vi "GESTIONE FRENO.vi"(10 "Sub Panel freno":refnum<vi>) -> ()   [LabVIEW 2019]
uses:
  TypeDef/InverterFreno.ctl
  TypeDef/Stato_inverter.ctl
  TypeDef/Comandi freno.ctl
  TypeDef/Stato inverter selezionato.ctl
  cDAQ_PLC Folder/cDAQ/SET SINGLE DO.ctl
  cDAQ_PLC Folder/cDAQ/DO List.ctl
  cDAQ_PLC Folder/cDAQ/SET SINGLE AO.ctl
  cDAQ_PLC Folder/cDAQ/AO List.ctl
  BenchSelector.vi
  Global_All_Data.vi
  Stato alimentatore 1.vi
  Global control type freno.vi
  Stato comandi freno.vi
  Global CAMBIO CTRL FRENO.vi
  Global FINE AVVIO.vi
  Fine rampa sinus penta.vi
  Global Trampa 0.vi
  Global CTRL VELOCITA.vi
  cDAQ_PLC Folder/cDAQ/SET ARRAY DO.ctl
  Global senso rotazione.vi
  <vilib>/Utility/file.llb/Read Delimited Spreadsheet (string).vi
panel:
  out "A max":dbl
  out "Freno selezionato":i32
  out "Rpm max":dbl
  out "Cmax":dbl
  out "KW max Banco 1":dbl
  out "KW max Banco 2":dbl
  out "RPM max Banco 1":dbl
  out "RPM max Banco 2":dbl
  out "A max Banco 2":dbl
  out "A max Banco 1":dbl
  out "Nm max Banco 2":dbl
  out "Nm max Banco 1":dbl
  out "all rows":string[][](array[string])
  out "Comandi freno":T1[](array[typedef]) {"Rif AO coppia freno[Nm]" format="%#_13g"}
  out "Array stato inverter freno":T1[](array[typedef]) {"Rif AO coppia freno[Nm]" format="%#_13g"}
  in  "rif vel":bool
  in  "Rif % AO RPM":dbl
  out "# elements in queue":i32
  out "DO senso rotaz freno":bool=TRUE
  out "Rpm stabile":bool
  out "Ctrl coppia":bool
  out "Ctrl velocità":bool
  in  "simula?":bool
  out "KW max banco":dbl
  out "Kw Max prova":dbl
  out "INVERTI SENSO ROT":bool
  out "DI senso rotaz freno":bool
  out "Message":string
  out "Abilita":bool=TRUE
  out "fine rampa C":bool
  out "fine rampa rpm":bool
  out "P Stabile?":bool
  out "start":bool=TRUE
  out "Controllo desiderato":T2(ring)
  out "Controllo effettivo":T2(ring)
  out "C Stabile?":bool
  out "Rif AO coppia freno [Nm]":dbl format="%#_13g"
  out "Rif AO vel [RPM]":dbl
  in  "Precisione pid Nm":dbl caption="Nm"
  in  "Precisione pid W":dbl caption="W"
  out "Boolean 2":bool
  in  "Compensazione velocità":bool=TRUE
  out "Comp.":bool
  in  "Gestione freno":T3 {"Status ref"."Speed" max=2000.0; "Status ref"."Torque" max=2000.0; "Control"."Set" min=0.0 max=0.0 format="%#.2f"}
  out "C->rpm":string
  out "rpm->C":string
  out "Boolean":bool
  in  "OK Button":bool
  out "Stato comandi":T3
  in  "Salva config freni":bool
  in  "rpm":dbl
  in  "x":dbl
  in  "stop":bool
  in  "ARRAY IMPOSTAZIONI INV.FRENI":T4[](array[typedef])=[{"Nome"="", "Cmax"=100.0, "Rpm max"=3000.0, "A max"=0.0, "Controllo RPM"={"PID gains Rpm"={"proportional gain (Kc)"=0.0, "integral time (Ti, min)"=0.0, "derivative time (Td, min)"=0.0}, "Abilita pid"=FALSE, "Precisione pid Rpm"=0.015, "Medie pid"=10, "Trampa[s]"=10, "Tstab ramp[s]"=10, "Max%pid"=10}, "Controllo coppia"={"PID gains Coppia"={"proportional gain (Kc)"=10.0, "integral time (Ti, min)"=0.015, "derivative time (Td, min)"=0.0}, "Abilita pid"=FALSE, "Precisione pid Nm"=0.0, "Medie pid"=0, "Trampa[s]"=0, "Tstab ramp[s]"=10, "Max%pid"=10}, "Controllo potenza"={"PID gains potenza"={"proportional gain (Kc)"=0.4, "integral time (Ti, min)"=0.025, "derivative time (Td, min)"=0.0}, "Abilita pid"=FALSE, "Precisione pid W"=0.015, "Medie pid"=10, "Trampa[s]"=10, "Tstab ramp[s]"=10, "Max%pid"=10}, "Compensa coppia residua"={"Abilita compensazione"=FALSE, "C residua [Nm]"=0.0, "C isteresi [Nm]"=0.0, "PID gains C-RPM"={"proportional gain (Kc)"=1.0, "integral time (Ti, min)"=0.01, "derivative time (Td, min)"=0.0}, "C precision [Nm]"=0.0, "Max%pid"=0, "Medie pid"=0}}, {"Nome"="", "Cmax"=200.0, "Rpm max"=4500.0, "A max"=0.0, "Controllo RPM"={"PID gains Rpm"={"proportional gain (Kc)"=0.0, "integral time (Ti, min)"=0.0, "derivative time (Td, min)"=0.0}, "Abilita pid"=FALSE, "Precisione pid Rpm"=0.015, "Medie pid"=10, "Trampa[s]"=10, "Tstab ramp[s]"=10, "Max%pid"=10}, "Controllo coppia"={"PID gains Coppia"={"proportional gain (Kc)"=10.0, "integral time (Ti, min)"=0.015, "derivative time (Td, min)"=0.0}, "Abilita pid"=FALSE, "Precisione pid Nm"=0.0, "Medie pid"=0, "Trampa[s]"=0, "Tstab ramp[s]"=10, "Max%pid"=10}, "Controllo potenza"={"PID gains potenza"={"proportional gain (Kc)"=0.4, "integral time (Ti, min)"=0.025, "derivative time (Td, min)"=0.0}, "Abilita pid"=FALSE, "Precisione pid W"=0.015, "Medie pid"=10, "Trampa[s]"=10, "Tstab ramp[s]"=10, "Max%pid"=10}, "Compensa coppia residua"={"Abilita compensazione"=FALSE, "C residua [Nm]"=0.0, "C isteresi [Nm]"=0.0, "PID gains C-RPM"={"proportional gain (Kc)"=1.0, "integral time (Ti, min)"=0.01, "derivative time (Td, min)"=0.0}, "C precision [Nm]"=0.0, "Max%pid"=0, "Medie pid"=0}}] {"Controllo RPM"."Precisione pid Rpm" format="%#_13g"; "Controllo RPM"."PID gains Rpm"."derivative time (Td, min)" format="%.3f"; "Controllo RPM"."PID gains Rpm"."integral time (Ti, min)" format="%.3f"; "Controllo RPM"."PID gains Rpm"."proportional gain (Kc)" format="%.3f"; "Controllo potenza"."Precisione pid W" format="%#_13g"; "Controllo potenza"."PID gains potenza"."derivative time (Td, min)" format="%.3f"; "Controllo potenza"."PID gains potenza"."integral time (Ti, min)" format="%.3f"; "Controllo potenza"."PID gains potenza"."proportional gain (Kc)" format="%.3f"; "Controllo coppia"."Precisione pid Nm" format="%#_13g"; "Controllo coppia"."PID gains Coppia"."derivative time (Td, min)" format="%.3f"; "Controllo coppia"."PID gains Coppia"."integral time (Ti, min)" format="%.3f"; "Controllo coppia"."PID gains Coppia"."proportional gain (Kc)" format="%.3f"; "Compensa coppia residua"."PID gains C-RPM"."derivative time (Td, min)" format="%.3f"; "Compensa coppia residua"."PID gains C-RPM"."integral time (Ti, min)" format="%.3f"; "Compensa coppia residua"."PID gains C-RPM"."proportional gain (Kc)" format="%.3f"}
  out "Numeric":i32
  in  "EXIT":bool
  in  "Letture":cluster{"RPM":dbl, "COPPIA":dbl, "POTENZA":dbl}
  # "CHANGING CONTROL\nTYPE...."
  # "CHANGING CONTROL\nTYPE...."
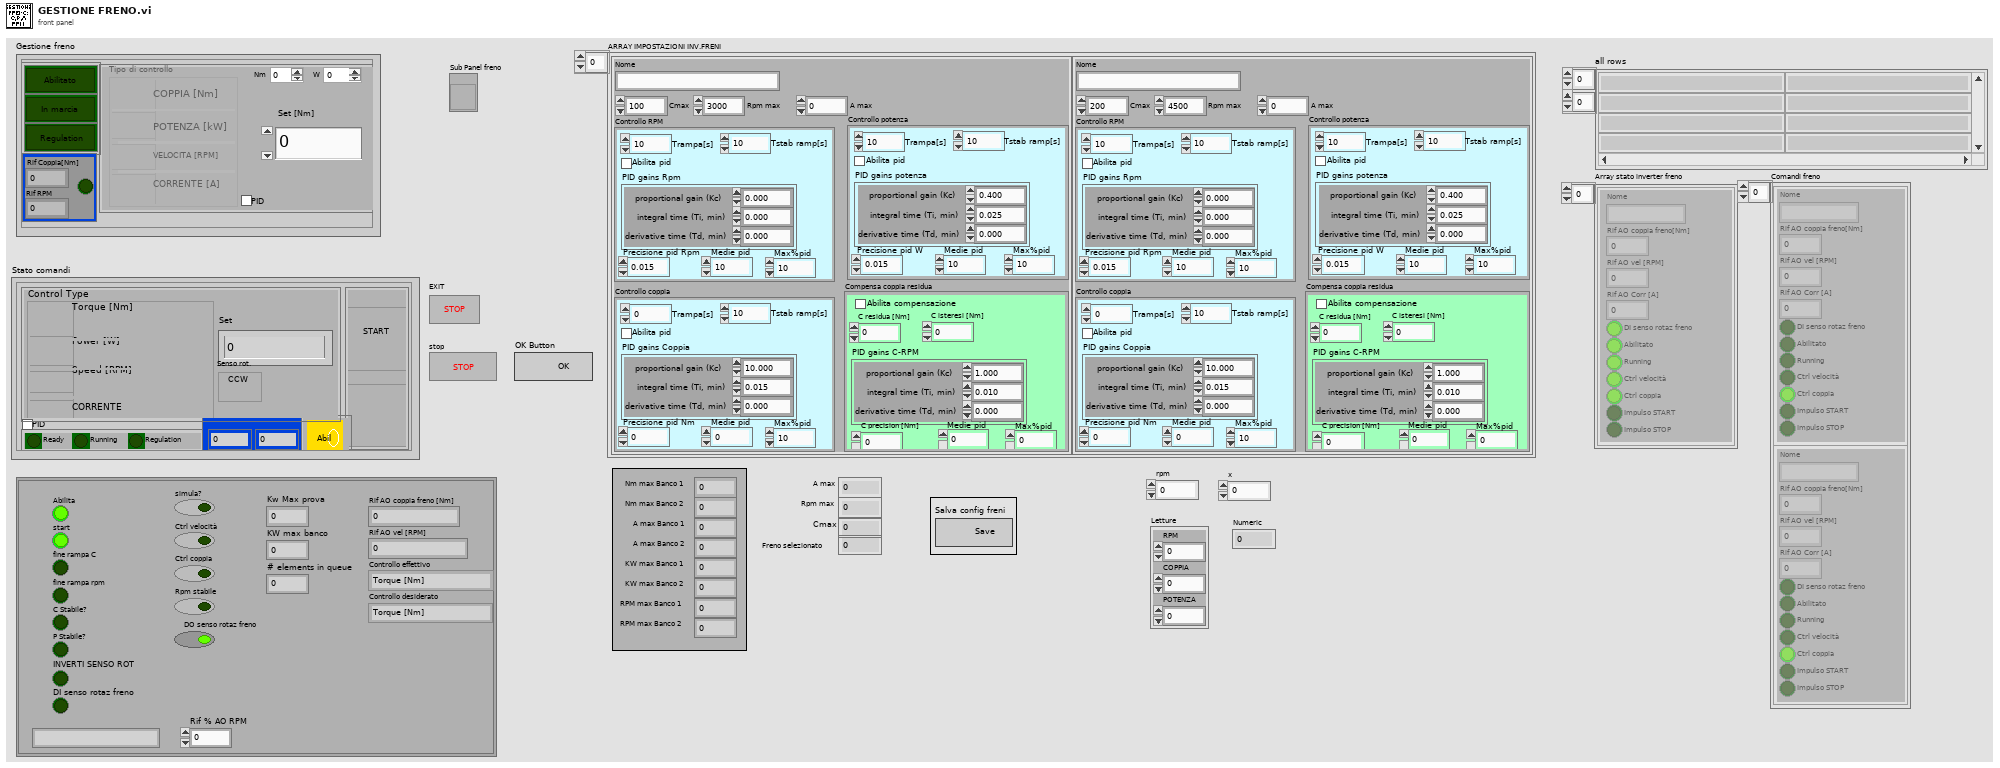
[diagram p1: front panel]
types:
  T1 = typedef "Stato_inverter.ctl" = cluster{"DI senso rotaz freno":bool, "Rif AO vel [RPM]":dbl, "Rif AO coppia freno[Nm]":dbl, "Abilitato":bool, "Running":bool, "Ctrl velocità":bool, "Nome":string, "Ctrl coppia":bool, "Impulso START":bool, "Impulso STOP":bool, "Rif AO Corr [A] ":dbl}
  T2 = enum32{"Torque [Nm]", "Power [W]", "Speed [RPM]", "Corrente [A]"}
  T3 = typedef "Comandi freno.ctl" = cluster{"Control":cluster{"Control Type":enum32{"Torque [Nm]", "Power [W]", "Speed [RPM]", "Corrente [A]"}, "Set":dbl, "Inverti senso di rotazione":bool}, "Start\\stop":cluster{"Start":bool, "STOP":bool}, "Status":cluster{"Ready":bool, "Running":bool, "Regulation":bool}, "PID":bool, "Abilita":cluster{"Abilita":bool}, "Status ref":cluster{"Torque":dbl, "Speed":dbl}}
  T4 = typedef "InverterFreno.ctl" = cluster{"Nome":string, "Cmax":dbl, "Rpm max":dbl, "A max":dbl, "Controllo RPM":cluster{"PID gains Rpm":cluster{"proportional gain (Kc)":dbl, "integral time (Ti, min)":dbl, "derivative time (Td, min)":dbl}, "Abilita pid":bool, "Precisione pid Rpm":dbl, "Medie pid":i32, "Trampa[s]":i32, "Tstab ramp[s]":i32, "Max%pid":i32}, "Controllo coppia":cluster{"PID gains Coppia":cluster{"proportional gain (Kc)":dbl, "integral time (Ti, min)":dbl, "derivative time (Td, min)":dbl}, "Abilita pid":bool, "Precisione pid Nm":dbl, "Medie pid":i32, "Trampa[s]":i32, "Tstab ramp[s]":i32, "Max%pid":i32}, "Controllo potenza":cluster{"PID gains potenza":cluster{"proportional gain (Kc)":dbl, "integral time (Ti, min)":dbl, "derivative time (Td, min)":dbl}, "Abilita pid":bool, "Precisione pid W":dbl, "Medie pid":i32, "Trampa[s]":i32, "Tstab ramp[s]":i32, "Max%pid":i32}, "Compensa coppia residua":cluster{"Abilita compensazione":bool, "C residua [Nm]":dbl, "C isteresi [Nm]":dbl, "PID gains C-RPM":cluster{"proportional gain (Kc)":dbl, "integral time (Ti, min)":dbl, "derivative time (Td, min)":dbl}, "C precision [Nm]":dbl, "Max%pid":i32, "Medie pid":i32}}
  T5 = cluster{"Message":string, "Message Data":variant}
  T6 = typedef "Stato inverter selezionato.ctl" = cluster{"Stato comandi freno":T3, "Stato":cluster{"rif C%":dbl, "rif vel%":dbl, "Controllo effettivo":enum32{"Torque [Nm]", "Power [W]", "Speed [RPM]"}, "Controllo desiderato":enum32{"Torque [Nm]", "Power [W]", "Speed [RPM]"}, "Fine rampa C":bool, "Fine rampa RPM":bool, "Senso rotaz":bool, "Start":bool, "C stabile":bool, "P stabile":bool, "RPM stabile":bool}}
  T7 = typedef "SET SINGLE DO.ctl" = cluster{"DO":T8, "Value":bool}
  T8 = typedef "DO List.ctl" = enum16{"OFF: ALL DO", "*ABILITA freno 1", "*ABILITA freno 2", "*ABILITA freno 3", "*START freno 1", "*START freno 2", "*START freno 3", "*STOP freno 1", "*STOP freno 3", "*STOP freno 2", "*Senso rot freno 1", "*Senso rot freno 2", "*Senso rot freno 3", "*Ctrl velocità freno 1", "*Ctrl velocità freno 2", "*Ctrl velocità freno 3", "*Ctrl coppia freno 1", "*Ctrl coppia freno 2", "*Ctrl coppia freno 3", "*ABILITA alimentatore 1", "*ABILITA alimentatore 2", "*ABILITA alimentatore 3", "*ABILITA alimentatore 4", "*START alimentatore 1", "*START alimentatore 2", "*START alimentatore 3", "*START alimentatore 4", "*STOP alimentatore 1", "*STOP alimentatore 2", "*STOP alimentatore 3", "*STOP alimentatore 4", "SENSO ROT alimentatore 1", "SENSO ROT alimentatore 2", "Abilita LEM 1000A", "Abilita LEM 300A", "Abilita sensori EXT WT", "B1 Seleziona linea 1", "B1 Seleziona linea 2", "B1 Seleziona linea 3", "B1 Seleziona linea 4", "B1 Seleziona linea 5", "B2 Seleziona linea 1", "B2 Seleziona linea 2", "B2 Seleziona linea 3", "B2 Seleziona linea 4", "B2 Seleziona linea 5", "*Reset allarmi", "*Start potenza AC", "*Stop potenza AC", "*Start potenza DC", "*Stop potenza DC", "*Start potenza DC eccit", "*Stop pontenza DC eccit", "Bypass res meter", "2nd canale res meter", "Enable res meter", "*Abilit teler ramo WT", "*Abil teler ramo princ Resit", "*Abil teler ramo 1 Resist", "*Abil teler ramo 2 Resist", "*Abil teler ramo 3 Resist", "*Abil cortocirc avvolgim", "*Controllo torsiometro B1", "*Controllo Torsiom B2", "*Scala torsiometro B1", "*Scala torsiometro B2", "*Collaudo in corso", "*Allarme presente", "Abilitazione elettroserratura", "Exit", "*Abilita collaudo", "*Abilita potenza trifase", "*Abilita potenza monofase", "*Abilita potenza DC", "*Abilita potenza DC eccit", "*Disabilita teleruttori potenza", "Set teleruttori prova a freddo", "Prova a freddo monofase", "Watchdog", "Forza DO PLC 3", "Forza DO PLC 2", "Forza DO PLC 1", "Forza DO cDAQ", "Scala 2000(T) 200(F) res meter", "Seleziona banco 1", "Seleziona banco 2", "Comando azionam in blocco", "Comando azionam reset", "Sensibilità freno 16 32 nm", "Reset Allarmi", "Carico res - Ramo 1", "Carico res - Ramo 2", "Carico res - Ramo 3", "Carico res - Ramo 4", "Carico res - Ramo 5", "Carico res - Ramo 6", "Carico res - Ramo 7", "Carico res - Ramo 8", "Carico res - Ramo 9", "Carico res - Ramo 10", "Carico res - Ramo 11", "Carico res - Start ventilatore", "Carico res - Stop ventilatore", "Abilita potenza solo freno", "Abilita AFE + freno trasc", "Abilita potenza carico resistivo", "Chiudi potenza AFE", "Apri potenza AFE", "Start AFE", "Config Banco2 TDE", "Misura diretto WT", "Ripristina centralina protezioni", "Abilita Scrittura Dati Keb", "Bench Selection(0-B1,1-B2)", "Select current mode", "Select torque mode", "Select speed mode", "Extenal alarm", "Enable Extenal program ", "Start ", "Stop", "Enable force mode", "Abilita linea 125 A", "Abilita linea 63 A", "Abilita linea 16 A", "Aum Tensione Variac", "Dim Tesnione Variac", "Abilita Ellecto Stractura", "Riprinto Emergenxe ", "Abilita Collaudo", "Disabilita Collaudo", "Abilita Ingresso Variac", "Abilita Uscita Variac", "Abilita ventilatore Variac"}
  T9 = typedef "SET SINGLE AO.ctl" = cluster{"AO":T10, "Value":dbl}
  T10 = typedef "AO List.ctl" = enum16{"OFF: ALL AO", "RIF VEL FRENO 1", "RIF VEL FRENO 2", "RIF VEL FRENO 3", "RIF COPPIA FRENO", "RIF COPPIA FRENO 1", "RIF COPPIA FRENO 2", "RIF COPPIA FRENO 3", "RIF CORRENTE FRENO 2", "RIF V ALIM 1", "RIF F ALIM 1", "RIF V ALIM 2", "RIF F ALIM 2", "RIF V ALIM 3", "RIF F ALIM 3", "RIF V ALIM 4", "RIF F ALIM 4", "FORZA AO PLC 3", "FORZA AO PLC 2", "FORZA AO PLC 1", "FORZA AO cDAQ", "Configura alimentatore keb", "Tempo rampa keb", "Condensatori", "Exit"}
  T11 = typedef "Cluster MISURE.ctl" = cluster{"MISURE NM":T12, "MISURE ALL":T13}
  T12 = typedef "MISURE NM.ctl" = cluster{"Banco":string, "Anno":string, "Numero":string, "Ntabella":string, "Misura":string, "Tipo Prova":string, "ProgressivoAcq":string, "Descrizione":string, "Data_ora":string, "t. acq [h:m:s]":string, "t. acq [min]":string, "t. acq [s]":string, "n [rpm]":string, "f [Hz]":string, "U1[V]":string, "U2 [V]":string, "U3 [V]":string, "U123_media [V]":string, "I1[A]":string, "I2[A]":string, "I3[A]":string, "I123_media [A]*I":string, "I_123_sbil [%]":string, "Ulin[V]":string, "Uc [V]":string, "Uaux [V]":string, "Ilin[A]*I":string, "Imar[A]":string, "Iaux[A]":string, "Uarm[V]":string, "Uecc[V]":string, "Iarm[A]*I":string, "Iecc[A]":string, "pf":string, "P1 [W]":string, "P1 [kW]":string, "Q [VAR]":string, "Q [kVAR]":string, "S [VA]":string, "S [kVA]":string, "P1arm[W]":string, "P1ecc[W]":string, "Parm[kW]":string, "P1ecc[kW]":string, "Cond[uF]":string, "P1_linea_6fili[W]":string, "P1_linea_6fili[kW]":string, "eta_gr_6fili [%]":string, "eta_inverter_6fili [%]":string, "pf_linea_6fili":string, "U4 [V]":string, "U5 [V]":string, "U6 [V]":string, "U456_media [V]":string, "I4 [A]":string, "I5 [A]":string, "I6 [A]":string, "I456_media [A]":string, "C [Nm]*C":string, "Cric [Nm]":string, "Cric\\Cnom":string, "Iric[A]":string, "Iric\\Inom":string, "P2_mecc [W]":string, "P2_mecc [kW]":string, "eta motore [%]":string, "Scorr[%]":string, "Tamb[°C]":string, "R1[ohm]":string, "R2[ohm]":string, "R3[ohm]":string, "Rmedia[ohm]":string, "DT_R1[°C]":string, "DT_R2[°C]":string, "DT_R3[°C]":string, "DT_media[°C]":string, "R_marcia[ohm]":string, "R_aux[ohm]":string, "DT_marcia[°C]":string, "DT_aux[°C]":string, "R_Arm[ohm]":string, "R_Ecc[ohm]":string, "DT_Arm[°C]":string, "DT_Ecc[°C]":string, "TambFreddo[°C]":string, "R1_freddo[ohm]":string, "R2_freddo[ohm]":string, "R3_freddo[ohm]":string, "Rmedia_freddo[ohm]":string, "R_Marcia_freddo[ohm]":string, "R_Aux_freddo[ohm]":string, "R_Arm_freddo[ohm]":string, "R_Ecc_freddo[ohm]":string, "TC1 [°C]":string, "TC2 [°C]":string, "TC3 [°C]":string, "TC4 [°C]":string, "TC5 [°C]":string, "TC6 [°C]":string, "TC7 [°C]":string, "TC8 [°C]":string, "PT1000_1[°C]":string, "PT1000_2[°C]":string, "PT1000_3[°C]":string, "Vdc eccitatrice[V]":string, "Idc eccitatrice[A]":string, "Vdc rotore[V]":string, "Idc rotore[A]":string, "Vac rotore[V]":string, "Iac rotore[V]":string, "V dinamo[V]":string, "Portata Q":string, "Pressione H":string, "U1'[V]":string, "U2'[V]":string, "U3'[V]":string, "I1'[A]":string, "I2'[A]":string, "I3'[A]":string, "U''R-N":string, "U''S-N":string, "U'' T-N":string, "U''R-S":string, "U''R-T":string, "U''S-T":string, "I1''[A]":string, "I2''[A]":string, "I3''[A]":string, "F''[Hz]":string, "P''[kW]":string, "CosFi''":string, "PT1000_4[°C]":string, "Scorta 3":string}
  T13 = typedef "Cluster misure ALL.ctl" = cluster{"Cluster READ NI":T14, "MISURE WT":T17, "Resistenze Resistomat":T18, "INTERFACCIA":T19, "FREDDO resistomat":cluster{"Res Ch1":dbl, "Res Ch2":dbl, "tAMB":dbl, "Res Ch3":dbl}, "STATO PLC 1":T24, "Res Ch2":dbl, "Res Ch2 2":dbl, "FREDDO res meter":cluster{"Res Ch1":dbl, "Res Ch2":dbl, "tAMB":dbl, "Res Ch3":dbl}, "Resistenze Res Meter":T18, "READ SINUS PENTA":T28, "STATO PLC 2":T29, "STATO PLC 3":T33, "DCREG":T37}
  T14 = typedef "Cluster NI.ctl" = cluster{"AI (0-10V)":cluster{"AI 0":dbl, "AI 1":dbl, "AI 2":dbl, "AI 3":dbl, "AI 4":dbl, "AI 5":dbl, "AI 6":dbl, "AI 7":dbl, "AI 8":dbl, "AI 9":dbl, "AI 10":dbl, "AI 11":dbl, "AI 12":dbl, "AI 13":dbl, "AI 14":dbl, "AI 15":dbl, "AI 16":dbl, "AI 17":dbl, "AI 18":dbl, "AI 19":dbl, "AI 20":dbl, "AI 21":dbl, "AI 22":dbl, "AI 23":dbl, "AI 24":dbl, "AI 25":dbl, "AI 26":dbl, "AI 27":dbl, "AI 28":dbl, "AI 29":dbl, "AI 30":dbl, "AI 31":dbl}, "StatoAO_Cdaq[0-10V]":cluster{"AO 1":dbl, "AO 2":dbl, "AO 3":dbl, "AO 4":dbl}, "Contatori [rpm]":cluster{"RPM 1":dbl, "RPM 2":dbl}, "StatoAO_Cdaq [4-20mA]":T15, "StatoDO_Cdaq":T16, "DI":cluster{"Scorta 0":bool, "Scorta 1":bool, "Scorta 2":bool, "Scorta 3":bool, "Scorta 4":bool, "Scorta 5":bool, "Scorta 6":bool, "Scorta 7":bool, "Scorta 8":bool, "Scorta 9":bool, "Scorta 10":bool, "Scorta 11":bool, "Scorta 12":bool, "Scorta 13":bool, "Scorta 14":bool, "Scorta 15":bool, "Scorta 16":bool, "Scorta 17":bool, "Scorta 18":bool, "Scorta 19":bool, "Scorta 20":bool, "Scorta 21":bool, "Scorta 22":bool, "Scorta 23":bool, "Scorta 24":bool, "Scorta 25":bool, "Scorta 26":bool, "Scorta 27":bool, "Scorta 28":bool, "Scorta 29":bool, "Scorta 30":bool, "Scorta 31":bool}, "AI (4-20mA)":cluster{"AI 0":dbl, "AI 1":dbl, "AI 2":dbl, "AI 3":dbl, "AI 4":dbl, "AI 5":dbl, "AI 6":dbl, "AI 7":dbl, "AI 8":dbl, "AI 9":dbl, "AI 10":dbl, "AI 11":dbl, "AI 12":dbl, "AI 13":dbl, "AI 14":dbl, "AI 15":dbl}, "TC [°C]":cluster{"tc 1":dbl, "tc 2":dbl, "tc 3":dbl, "tc 4":dbl}, "NI Read Values":cluster{"RPM":dbl, "Frequency":dbl, "Mod 1":cluster{"Torsiometro 1":dbl, "Torsiometro 2":dbl, "Strin Gauge 1":dbl, "Strin Gauge 2":dbl}, "Mod 2":cluster{"Termocoppia 1":dbl, "Termocoppia 2":dbl, "Termocoppia 3":dbl, "Termocoppia 4":dbl}, "Mod 3":cluster{"PT 100 1":dbl, "PT 100 2":dbl, "PT 100 3":dbl, "PT 100 4":dbl}}}
  T15 = typedef "StatoAO_cdaq.ctl" = cluster{"Cdaq_AO [0-10V] 0 for Torque":dbl, "Cdaq_AO [0-10V] 1":dbl, "Cdaq_AO [0-10V] 2":dbl, "Cdaq_AO [0-10V] 3":dbl}
  T16 = typedef "statoDO_Cdaq.ctl" = cluster{"Scorta 0":bool, "Scorta 1":bool, "Scorta 2":bool, "Scorta 3":bool, "Scorta 4":bool, "Scorta 5":bool, "Scorta 6":bool, "Scorta 7":bool, "Scorta 8":bool, "Scorta 9":bool, "Scorta 10":bool, "Scorta 11":bool, "Scorta 12":bool, "Scorta 13":bool, "Scorta 14":bool, "Scorta 15":bool, "Scorta 16":bool, "Scorta 17":bool, "Scorta 18":bool, "Scorta 19":bool, "Scorta 20":bool, "Scorta 21":bool, "Scorta 22":bool, "Scorta 23":bool, "Scorta 24":bool, "Scorta 25":bool, "Scorta 26":bool, "Scorta 27":bool, "Scorta 28":bool, "Scorta 29":bool, "Scorta 30":bool, "Scorta 31":bool}
  T17 = typedef "MISURE WT.ctl" = cluster{"URMS 1":dbl, "IRMS 1":dbl, "P 1":dbl, "S 1":dbl, "Q 1":dbl, "LAMBDA 1":dbl, "PHI 1":dbl, "F U 1":dbl, "F I 1":dbl, "NONE 1":dbl, "URMS 2":dbl, "IRMS 2":dbl, "P 2":dbl, "S 2":dbl, "Q 2":dbl, "LAMBDA 2":dbl, "PHI 2":dbl, "F U 2":dbl, "F I 2":dbl, "NONE 2":dbl, "URMS 3":dbl, "IRMS 3":dbl, "P 3":dbl, "S 3":dbl, "Q 3":dbl, "LAMBDA 3":dbl, "PHI 3":dbl, "F U 3":dbl, "F I 3":dbl, "NONE 3":dbl, "URMS SIGMA":dbl, "IRMS SIGMA":dbl, "P SIGMA":dbl, "S SIGMA":dbl, "Q SIGMA":dbl, "LAMBDA SIGMA":dbl, "PHI SIGMA":dbl, "F U SIGMA":dbl, "F I SIGMA":dbl, "NONE 4":dbl}
  T18 = typedef "ClusterRes.ctl" = cluster{"Res Ch1":dbl, "Res Ch2":dbl, "Res Ch3":dbl, "Tamb":dbl}
  T19 = typedef "INTERFACCIA.ctl" = cluster{"AI":cluster{"Portate":T20[], "Pressioni":T20[], "Coppie[Nm]":T20[], "Valvole prop %":T20[], "RPM":T20[], "Livelli":T20[], "Temperature":T20[], "Riferimenti %":T20[], "TENSIONI":T20[], "CORRENTI":T20[]}, "DI (logici)":cluster{"Start da pulsantiera":bool, "Stop da pulsantiera":bool, "Reset da pulsantiera":bool, "Sistema OK":bool, "Collaudo abilitato":bool, "Potenza trifase abilitata":bool, "Potenza monofase abilitata":bool, "Potenza DC abilitata":bool, "Potenza DC ECC abilitata":bool, "Start alimentazione AC":bool, "Start alimentazione DC":bool, "Start DC eccitazione":bool, "Teleruttore WT abilitato":bool, "Teleruttore Resistomat abilitato":bool, "Teleruttore corto fasi":bool, "Ramo 1 resistomat":bool, "Ramo 2 resistomat":bool, "Ramo 3 resistomat":bool, "B1 Scelta linea elettrica 1":bool, "B1 Scelta linea elettrica 2":bool, "B1 Scelta linea elettrica 3":bool, "B1 Scelta linea elettrica 4":bool, "B1 Scelta linea elettrica 5":bool, "B2 Scelta linea elettrica 1":bool, "B2 Scelta linea elettrica 2":bool, "B2 Scelta linea elettrica 3":bool, "B2 Scelta linea elettrica 4":bool, "B2 Scelta linea elettrica 5":bool, "Rotore bloccato 1":bool, "Rotore bloccato 2":bool, "FRENO 1 abilitato":bool, "FRENO 1 run":bool, "FRENO 1 senso rotaz":bool, "FRENO 1 ctrl velocità":bool, "FRENO 2 abilitato":bool, "FRENO 2 run":bool, "FRENO 2 senso rotaz":bool, "FRENO 2 ctrl velocità":bool, "ALIM 1 abilitato":bool, "ALIM 1 run":bool, "ALIM 2 abilitato":bool, "ALIM 2 run":bool, "ALIM 3 abilitato":bool, "ALIM 3 run":bool, "FRENO 1 ctrl coppia":bool, "FRENO 2 ctrl coppia":bool, "FRENO 3 ctrl coppia":bool, "DI (logici) aggiuntivi impianto":cluster{"Solo freno abilitato":bool, "Carico resistivo abilitato":bool, "AFE+freno abilitato":bool, "Protezioni chiuse":bool, "Start potenza AFE":bool, "AFE in marcia":bool}, "Misura corrente diretta WT":bool, "Misura corrente sens ext":bool, "Sens ext abilitati":bool}, "AO non scalati":T22, "AO scalati":T22, "DO (logici)":T23}
  T20 = typedef "ClusterMisura_e_Unità_INPUT.ctl" = cluster{"Misura":dbl, "UM":T21, "Descrizione":string}
  T21 = typedef "UnitàMisura.ctl" = enum16{"V", "mA", "Bar", "RPM", "m3/s", "m3/min", "m3/h", "l/s", "l/min", "in3/min", "ft3/min", "gpm", "igpm", "igph", "%", "°C", "m", "Nm", "A"}
  T22 = typedef "Lista AO sistema.ctl" = cluster{"FRENO1 rif vel":dbl, "FRENO1 rif Coppia":dbl, "FRENO2 rif vel":dbl, "FRENO2 rif Coppia":dbl, "ALIM1 rif V":dbl, "ALIM1 rif F":dbl, "ALIM2 rif V":dbl, "ALIM2 rif F":dbl, "ALIM3 rif V":dbl, "ALIM3 rif F":dbl, "Fnom keb":dbl, "Rpm nom keb":dbl, "Pnom keb":dbl, "Inom keb":dbl, "Vnom keb":dbl, "Rpm max keb":dbl, "Tempo rampa keb":dbl, "Tipo Mot keb":dbl, "FRENO  rif Coppia ":dbl, "FRENO  rif  Corrente":dbl}
  T23 = typedef "DOinterfaccia.ctl" = cluster{"Scelta banco 1":bool, "Scelta banco 2":bool, "Scelta banco 3":bool, "FRENO 1 abilita":bool, "FRENO 1 start":bool, "FRENO 1 senso rotaz":bool, "FRENO 1 ctrl velocità":bool, "FRENO 2 abilita":bool, "FRENO 2 start":bool, "FRENO 2 senso rotaz":bool, "FRENO 2 ctrl velocità":bool, "ALIM 1 abilita":bool, "ALIM 1 start":bool, "ALIM 2 abilita":bool, "ALIM 2 start":bool, "ALIM 3 abilita":bool, "ALIM 3 start":bool, "Abilita linea trifase":bool, "Abilita linea monofase":bool, "Abilita linea dc":bool, "Abilita linea dc eccit":bool, "B1 Linea elettrica 1":bool, "B1 Linea elettrica 2":bool, "B1 Linea elettrica 3":bool, "B1 Linea elettrica 4":bool, "B1 Linea elettrica 5":bool, "B2 Linea elettrica 1":bool, "B2 Linea elettrica 2":bool, "B2 Linea elettrica 3":bool, "B2 Linea elettrica 4":bool, "B2 Linea elettrica 5":bool, "Start potenza AC":bool, "Stop pontenza AC":bool, "Start potenza DC":bool, "Stop potenza DC":bool, "Start potenza eccitaz":bool, "Stop potenza eccitaz":bool, "Reset allarmi":bool, "watchdog":bool, "Scala torsiometro B1":bool, "Controllo torsiom B1":bool, "Scala torsiometro B2":bool, "Controllo torsiom B2":bool, "Teleruttore WT abilita":bool, "Teleruttore Resistomat abilita":bool, "Teleruttore corto fasi":bool, "Ramo 1 resistomat":bool, "Ramo 2 resistomat":bool, "Ramo 3 resistomat":bool, "Collaudo in corso":bool, "Allarme presente":bool, "Enable Res Meter":bool, "Bypass Res Meter":bool, "2nd canale Res Meter":bool, "Scala 200/2000 res meter":bool, "Taratura res meter":bool, "FRENO 1 ctrl coppia":bool, "FRENO 2 ctrl coppia":bool, "FRENO 3 ctrl coppia":bool, "Aggiuntivi impianto":cluster{"Senso rotazione alim 1":bool, "Senso rotazione alim 2":bool}, "ALIM 1 stop":bool, "ALIM 2 stop":bool, "ALIM 3 stop":bool, "FRENO 1 stop":bool, "FRENO 2 stop":bool, "FRENO 3 stop":bool, "B1 configurazione freno B":bool, "B2 configurazione freno B":bool, "Abilita scrittura KEB":bool, "Bench Selection (0-B1,1-B2)":bool, "Select current mode":bool, "Select torque mode":bool, "Select speed mode":bool, "Start":bool, "Stop":bool, "Block":bool, "Enable Force mode":bool, "Abilita linea 125 A":bool, "Abilita linea 63 A":bool, "Abilita linea 16 A":bool, "Aum Tensione Variac":bool, "Dim Tesnione Variac":bool, "Abilita ellectro stractura":bool, "Risprinito Emergence":bool, "Abilita collaudo":bool, "Disabilita collaudo":bool, "External Alaram":bool, "Enable external program":bool, "Reset":bool, "Abilita Ingresso Variac":bool, "Abilita Ventilatore Variac":bool, "Abilita Uscita Variac ":bool}
  T24 = typedef "STATO PLC 1.ctl" = cluster{"USCITE PLC":T25, "Stato DI_PLC":cluster{"Sistema OK":bool, "Rotore bloccato":bool, "Scorta 1":bool, "Prova diretto inverter":bool, "Prova con filtro LC":bool, "Teleruttore WT abilitato":bool, "Alim sinus penta abilitato":bool, "Alim sinus penta in marcia":bool, "Freno abilitato":bool, "Freno in marcia":bool, "Senso rotazione freno":bool, "Potenza abilitata":bool, "Scorta 3":bool, "Scorta 4":bool, "scorta 5":bool, "scorta 6":bool}, "AI plc":cluster{"Allarmi 1":dbl, "Allarmi 2":dbl, "Scorta 1":dbl, "Scorta 2":dbl, "RPM mot prova":dbl, "I mot prova":dbl, "RPM freno":dbl, "I freno":dbl, "Scorta 3":dbl, "Scorta 4":dbl}}
  T25 = typedef "Uscite PLC 1.ctl" = cluster{"AO (real) 2":cluster{"SCORTA 1":dbl, "SCORTA 2":dbl, "SCORTA 3":dbl, "SCORTA 4":dbl, "SCORTA 5":dbl, "SCORTA 6":dbl, "SCORTA 7":dbl, "SCORTA 8":dbl}, "statoAO_PLC out":T26, "DO (bit)":T27}
  T26 = typedef "statoAO_plc_1.ctl" = cluster{"Rif Lim coppia freno [%]":dbl, "Rif rpm freno [%]":dbl, "Rif coppia freno [%]":dbl, "Rif V alimentatore [%]":dbl, "Rif F alimentatore [%]":dbl}
  T27 = typedef "StatoDO_PLC_1.ctl" = cluster{"Scelta banco 1":bool, "Set dati motore freno 2":bool, "Diretto inverter":bool, "Filtro LC":bool, "Marcia ALIM (1s)":bool, "Marcia FRENO (1s)":bool, "Stop AFE (1s)":bool, "Stop freno (1s)":bool, "Reset allarmi":bool, "Watchdog":bool, "Senso rotazione":bool, "Abilita collaudo (1s)":bool, "Disabilita collaudo (1s)":bool, "Abilitazione ALIM":bool, "Abilitazione FRENO":bool, "Teleruttore WT":bool, "Senso rot motore prova":bool, "Scorta 7":bool, "Scorta 8":bool, "Scorta 9":bool, "Scorta 10":bool, "Scorta 11":bool, "Scorta 12":bool, "Scorta 13":bool}
  T28 = typedef "Parametri inverter letti.ctl" = cluster{"Menù Misure motore (M000-M030)":cluster{"Rif vel a regime (int)":u16, "Rif vel a regime (dec)":u16, "Rif vel dopo rampe (int)":u16, "Rif vel dopo rampe (dec)":u16, "RPM motore (int)":u16, "RPM motore (dec)":u16, "FREQout inverter":u16, "Rif coppia a regime(Nm)":u16, "Richiesta di coppia (Nm)":u16, "Coppia generata dal motore(Nm)":u16, "Rif coppia a regime(%)":u16, "Richiesta di coppia (%)":u16, "Coppia generata dal motore(%)":u16, "Coppia max richiesta prima delle rampe(Nm)":u16, "Coppia max richiesta dopo le rampe(Nm)":u16, "Limite di velocità prima delle rampe":u16, "Limite di velocità dopo le rampe":u16, "Coppia max richiesta prima delle rampe(%)":u16, "Coppia max richiesta dopo le rampe(%)":u16, "Rif di flusso":u16, "Corrente di uscita":u16, "Capacità termica del motore":u16, "Tensione di uscita":u16, "Potenza di uscita":u16, "Energia consumata (LSword)":u16, "Energia consumata (MSword)":u16, "Tensione bus DC":u16, "Tensione di rete":u16}, "Menù regolatore PID (M018-M024)":cluster{"Rif PID a regime(%)":u16, "Rif pid dopo rampe(%)":u16, "Retroazione del pid(%)":u16, "Errore del pid(%)":u16, "uscita del pid(%)":u16, "Rif del pid dopo le rampe":u16, "Retroazione del pid":u16}, "Menù ingressi digitali (M031-M036)":cluster{"Ingressi digitali ritardati":u16, "Ingressi digitali istantanei":u16, "Moresettiera comando loc":u16, "Morsett comando da seriale":u16, "Morsett comando bus di campo":u16, "Ing dig ausiliari da morsettiera":u16, "Ing dig ausiliari da seriale":u16}, "Menù riferimenti (M037-M051)":cluster{"Rif analog est REF":u16, "Rif analog est AIN1":u16, "Rif analog est AIN2":u16, "Rif analog est XAIN4":u16, "Rif analog est XAIN5":u16, "Rif velocità da seriale(int)":u16, "Rif velocità bus di campo(int)":u16, "Rif coppia da seriale":u16, "Rif coppia bus di campo":u16, "Rif del PID da seriale":u16, "Rif del PID da bus di campo":u16, "Retroazione del PID da seriale":u16, "Retroazione del PIDda bus di campo":u16, "Rif da encoder":u16, "Rif in frequenza":u16, "Rif velocità da seriale(dec)":u16, "Rif velocità bus di campo(dec)":u16}, "Menù rampe (P009-P033)":cluster{"Tempo di dec rampa di vel 1":u16, "Tempo di acc rampa di vel 2":u16, "Tempo di dec rampa di vel 2":u16, "Tempo di acc rampa di vel 1":u16, "Unità di mis tempi rampe vel 1/2":u16, "Tempo di acc rampa di vel 3":u16, "Tempo di dec rampa di vel 3":u16, "Tempo di acc rampa di vel 4":u16, "Tempo di dec rampa di vel 4":u16, "Unità di mis tempi rampe vel 3/4":u16, "Selettore arrottondam rampe":u16, "Tempo di arrotond iniz rampa acc":u16, "Tempo di arrotond finale rampa acc":u16, "Tempo di arrotond iniz rampa dec":u16, "Tempo di rampa di salita rif coppia":u16, "Tempo di rampa di discesa rif coppia":u16, "Unità di misura rampa coppia":u16, "Tempo rampa acc marcia jog":u16, "Tempo rampa dec marcia jog":u16, "Reset acc ai cambi pendenza":u16, "rampa di acc in fire mode":u16, "rampa di dec in fire mode":u16, "Tempo di arrotond finale rampa dec":u16}, "Menù controllo motore(C008-C128)":cluster{"Numero motori configurati":u16, "Tipo algoritmo di controllo Mot1":u16, "Tipo rif Mot1":u16, "Tensione nominale rete":u16, "Retroaz di vel da encoder Mot1":u16, "Tipo curva V/f Mot1":u16, "Rotazione delle fasi Mot1":u16, "Freq nominale del motore Mot1":u16, "RPM nominali del motore Mot1":u16, "Potenza nominale del motore Mot1":u16, "Corrente nominale del motore Mot1":u16, "Tensione nominale del motore mot1":u16, "Potenza a vuoto del motore Mot1":u16, "Corrente a vuoto del motore Mot1":u16, "Resistenza statorica del motore Mot1":u16, "Induttanza di dispersione Mot1":u16, "Induttanza mutua motore":u16, "Costante di tempo rotorica":u16, "Costante di tempo filtro pb":u16, "Velocità minima motore":u16, "Velocità massima motore":u16}, "Menù configurazione PID":cluster{"Selezione riferimento n.1":u16, "Selezione retroazione n.1":u16, "Modalità di fuzionamento PID":u16, "Termine derivativo calcolato su err o mis":u16, "Proporz moltiplica deriv e integrale":u16, "Azione del PID":u16}, "ID":dbl, "Menù uscite digitali":cluster{"MDO4 Inverter pronto":u16}, "Fcarrier":cluster{"Fcarrier Min (Hz)":u16, "Fcarrier Max (Hz)":u16}, "stato inverter M089":dbl, "Riferimenti":cluster{"Rif tensione":u16, "Rif velocità":u16}, "Comunicazione":bool, "Modalità stop":dbl}
  T29 = typedef "STATO PLC 2.ctl" = cluster{"USCITE PLC":T30, "Stato DI_PLC":cluster{"Sistema ok":bool, "Relè Resistomat abilitato":bool, "Freno abilitato":bool, "Freno in marcia":bool, "scorta b":bool, "scorta a":bool, "scorta 1":bool, "scorta 2":bool, "scorta 3":bool, "scorta 4":bool, "Scorta 5":bool, "Scorta 6":bool, "Scorta 7":bool, "Scorta 8":bool, "Scorta 9":bool, "Scorta 10":bool}, "AI plc":cluster{"Allarmi 1":dbl, "Allarmi 2":dbl, "TC 1":dbl, "TC 2":dbl, "TC 3":dbl, "TC 4":dbl, "TC 5":dbl, "TC 6":dbl, "TC 7":dbl, "TC 8":dbl, "PT1000 1":dbl, "PT1000 2":dbl, "PT1000 3":dbl, "PT1000 4":dbl}}
  T30 = typedef "Uscite PLC 2.ctl" = cluster{"AO (real) 2":cluster{"SCORTA 1":dbl, "SCORTA 2":dbl, "SCORTA 3":dbl, "SCORTA 4":dbl, "SCORTA 5":dbl, "SCORTA 6":dbl, "SCORTA 7":dbl, "SCORTA 8":dbl}, "statoAO_PLC out":T31, "DO (bit)":T32}
  T31 = typedef "statoAO_plc_2.ctl" = cluster{"Condensatori":dbl, "Scorta 1":dbl, "Scorta 2":dbl}
  T32 = typedef "StatoDO_PLC_2.ctl" = cluster{"Relè misura resistomat":bool, "Misura res ramo 1":bool, "Misura res ramo 2":bool, "Misura res ramo 3":bool, "Scelta banco 2":bool, "Scala Torsiometro":bool, "Ctrl torsiometro":bool, "Select current mode":bool, "Select Torque mode":bool, "Select speed mode":bool, "Watchdog":bool, "Scorta":bool, "Scorta 2":bool, "Scorta 3":bool, "Scorta 4":bool, "Scorta 5":bool, "Bench selection":bool, "External alarm":bool, "Enable external program":bool, "Reset allarmi":bool, "Start":bool, "Stop":bool, "Block":bool, "Scorta 6":bool}
  T33 = typedef "STATO PLC 3.ctl" = cluster{"USCITE PLC":T34, "Stato DI_PLC":cluster{"Sistema OK":bool, "Rotore bloccato":bool, "Filtro LC":bool, "Bypass Filtro LC":bool, "Scelta Trasformatore":bool, "Scelta Bypass trasformatore":bool, "Teleruttore wt abilitato":bool, "Alimentatore abilitato":bool, "Alimentatore in marcia":bool, "Scorta 1":bool, "Scorta 2":bool, "Scorta 3":bool, "Potenza abilitata":bool, "Alimentatore in allarme":bool, "Scorta 4":bool, "Conferma dati KEB":bool, "Scorta 5":bool, "Warning Inverter Alimentatore":bool, "Variac Abilitato":bool, "Linea 125 A abilitata":bool, "Linea 63 A abilitata":bool, "Linea 16 A abilitata":bool, "Scorta 6":bool, "Enable force mode":bool}, "AI plc":cluster{"Allarmi 1":dbl, "Allarmi 2":dbl, "RPM motore prova":dbl, "Corrente motore prova":dbl, "RPM freno":dbl, "Corrente freno":dbl, "Tipo motore keb":dbl, "I nom keb":dbl, "RPM nom keb":dbl, "V nom keb":dbl, "F nom keb":dbl, "T rampa keb":dbl, "scorta":dbl, "Scorta 2":dbl}}
  T34 = typedef "Uscite PLC 3.ctl" = cluster{"AO (real) 2":cluster{"SCORTA 1":dbl, "SCORTA 2":dbl, "SCORTA 3":dbl, "SCORTA 4":dbl, "SCORTA 5":dbl, "SCORTA 6":dbl, "SCORTA 7":dbl, "SCORTA 8":dbl}, "statoAO_PLC out":T35, "DO (bit)":T36}
  T35 = typedef "statoAO_plc_3.ctl" = cluster{"Rif velocità alimentatore":dbl, "Scorta":dbl, "Tipo Motore  keb":dbl, "I nom keb":dbl, "RPM nom keb":dbl, "V nom keb":dbl, "F nom keb":dbl, "t rampa keb":dbl}
  T36 = typedef "StatoDO_PLC_3.ctl" = cluster{"Select linea Inverter":bool, "Abilita sense wattmetro":bool, "Bypass filtro LC":bool, "Filtro LC":bool, "Bypass trasformatore":bool, "Trasformatore":bool, "Abilita uscite variac":bool, "Abilita linea 125 A":bool, "Abilita linea 63 A":bool, "Abilita linea 16 A":bool, "Abilita Scrittura Dati Keb":bool, "Abilita alimentatore":bool, "Marcia alimentatore (1s)":bool, "Stop alimentatore (1s)":bool, "Senso rot mot prova":bool, "Watchdog":bool, "Aumenta tensione variac":bool, "Diminuisci tensione variac ":bool, "Blocco elettroserrature":bool, "Ripristino emergence":bool, "Abilita ingresso variac":bool, "Abilita ventilatore variac":bool, "Reset Allarm":bool, "Scorta 1":bool, "Scorta 2":bool, "Scorta 3":bool, "Scorta 4":bool, "Scorta 5":bool, "Scorta 6":bool, "Scorta 7":bool, "Scorta 8":bool, "Scorta 9":bool, "Abilita collaudo":bool, "Disabilita collaudo ":bool, "Scorta 10":bool, "Scorta 11":bool, "Scorta 12":bool, "Scorta 13":bool, "Scorta 14":bool, "Scorta 15":bool}
  T37 = typedef "Parametri DCREG letti.ctl" = cluster{"Parametri di misura":cluster{"M000":dbl, "M001":dbl, "M002":dbl, "M003":dbl, "M004":dbl, "M005":dbl, "M006":dbl, "M007":dbl, "M008":dbl, "M009":dbl, "M010":dbl, "M011":dbl, "M012":dbl, "M013":dbl, "M014":dbl, "M015":dbl, "M016":dbl, "M017":dbl, "M018":dbl, "M019":dbl, "M020":dbl, "M021":dbl, "M022":dbl, "M023":dbl, "M024":dbl, "M025":dbl, "M026":dbl, "M027":dbl, "M028":dbl, "M029":dbl, "M030":dbl, "M031":dbl}, "Parametri di programmazione":cluster{"P000":dbl, "P001":dbl, "P002":dbl, "P003":dbl, "P004":dbl, "P005":dbl, "P006":dbl, "P010":dbl, "P011":dbl, "P012":dbl, "P013":dbl, "P014":dbl, "P015":dbl, "P016":dbl, "P030":dbl, "P031":dbl, "P032":dbl, "P033":dbl, "P034":dbl, "P035":dbl, "P036":dbl, "P037":dbl, "P038":dbl, "P039":dbl, "P040":dbl, "P050":dbl, "P051":dbl, "P052":dbl, "P053":dbl, "P054":dbl, "P055":dbl, "P056":dbl, "P057":dbl, "P058":dbl, "P059":dbl, "P060":dbl, "P061":dbl, "P062":dbl, "P070":dbl, "P071":dbl, "P073":dbl, "P074":dbl, "P076":dbl, "P077":dbl, "P079":dbl, "P080":dbl, "P082":dbl, "P083":dbl, "P084":dbl, "P085":dbl, "P086":dbl, "P087":dbl, "P088":dbl, "P100":dbl, "P101":dbl, "P102":dbl, "P103":dbl, "P104":dbl, "P110":dbl, "P111":dbl, "P120":dbl, "P121":dbl, "P122":dbl, "P123":dbl, "P124":dbl, "P125":dbl, "P126":dbl, "P127":dbl, "P128":dbl, "P129":dbl, "P130":dbl, "P131":dbl, "P132":dbl, "P133":dbl, "P134":dbl, "P150":dbl, "P151":dbl, "P152":dbl, "P153":dbl, "P154":dbl, "P155":dbl, "P156":dbl, "P157":dbl, "P158":dbl, "P170":dbl, "P171":dbl, "P172":dbl, "P173":dbl, "P174":dbl, "P175":dbl, "P176":dbl, "P177":dbl, "P178":dbl, "P179":dbl, "P180":dbl, "P181":dbl, "P182":dbl, "P183":dbl, "P184":dbl, "P185":dbl, "P186":dbl, "P187":dbl, "P188":dbl, "P189":dbl, "P190":dbl, "P191":dbl, "P192":dbl, "P193":dbl, "P194":dbl, "P195":dbl, "P196":dbl, "P197":dbl, "P198":dbl, "P199":dbl, "P211":dbl, "P212":dbl, "P213":dbl, "P214":dbl, "P215":dbl, "P216":dbl, "P217":dbl, "P221":dbl, "P222":dbl, "P223":dbl, "P224":dbl, "P230":dbl, "P231":dbl, "P240":dbl, "P250":dbl, "P251":dbl}, "Parametri di configurazione":cluster{"C000":dbl, "C001":dbl, "C002":dbl, "C010":dbl, "C011":dbl, "C012":dbl, "C014":dbl, "C015":dbl, "C016":dbl, "C017":dbl, "C018":dbl, "C030":dbl, "C050":dbl, "C051":dbl, "C052":dbl, "C060":dbl, "C061":dbl, "C062":dbl, "C063":dbl, "C070":dbl, "C072":dbl, "C074":dbl, "C090":dbl, "C091":dbl, "C092":dbl, "C093":dbl, "C094":dbl, "C100":dbl, "C101":dbl, "C102":dbl, "C103":dbl, "C105":dbl, "C106":dbl, "C107":dbl, "C108":dbl, "C110":dbl, "C111":dbl, "C112":dbl, "C120":dbl, "C121":dbl, "C122":dbl, "C130":dbl, "C131":dbl, "C132":dbl, "C133":dbl, "C134":dbl, "C135":dbl, "C141":dbl, "C142":dbl, "C143":dbl, "C150":dbl, "C151":dbl, "C153":dbl, "C154":dbl, "C155":dbl, "C156":dbl, "C157":dbl, "C158":dbl, "C159":dbl, "C160":dbl, "C161":dbl, "C162":dbl, "C163":dbl, "C164":dbl, "C165":dbl, "C170":dbl}, "Codice allarme":dbl, "Comunicazione":bool}
  T38 = cluster{"DI senso rotaz freno":bool, "Rif AO vel [RPM]":bool, "Rif AO coppia freno[Nm]":bool, "Abilitato":bool, "Running":bool, "Ctrl velocità":bool, "Nome":bool, "Ctrl coppia":bool, "Impulso START":bool, "Impulso STOP":bool, "Rif AO Corr [A] ":bool}
  T39 = typedef "Comandi_Alimentatore.ctl" = cluster{"RIF 1":dbl, "RIF 2":dbl, "Status":cluster{"Ready":bool, "Running":bool, "Regulation":bool}, "Start\\stop":cluster{"Start":bool, "Stop":bool}, "PID RIF1":bool, "PID RIF2":bool, "Status ref":cluster{"RIF 1":dbl, "RIF 2":dbl}, "Abilita":cluster{"Abilita":bool}}
  T40 = cluster{"RIF 1":dbl, "RIF 2":dbl, "Abilitato":bool, "In marcia":bool, "Fine rampa RIF1":bool, "Fine rampa RIF2":bool, "Vstabile":bool, "F stabile":bool, "PID RIF1":bool, "PID RIF2":bool, "Alimentatore 1":T39}
  T41 = enum16{"open", "replace", "create", "open or create", "replace or create", "replace or create with confirmation"}
  T42 = enum8{"Enabled", "Disabled", "Disabled and Grayed Out"}
  T43 = typedef "SET ARRAY DO.ctl" = T7[]
  T44 = enum32{"Torque [Nm]", "Power [W]", "Speed [RPM]"}
  T45 = cluster{"Abilita compensazione":bool, "C residua [Nm]":dbl, "C isteresi [Nm]":dbl, "PID gains C-RPM":cluster{"proportional gain (Kc)":dbl, "integral time (Ti, min)":dbl, "derivative time (Td, min)":dbl}, "C precision [Nm]":dbl, "Max%pid":i32, "Medie pid":i32}
  T46 = cluster{"PID gains Coppia":cluster{"proportional gain (Kc)":dbl, "integral time (Ti, min)":dbl, "derivative time (Td, min)":dbl}, "Abilita pid":bool, "Precisione pid Nm":dbl, "Medie pid":i32, "Trampa[s]":i32, "Tstab ramp[s]":i32, "Max%pid":i32}
  T47 = cluster{"PID gains potenza":cluster{"proportional gain (Kc)":dbl, "integral time (Ti, min)":dbl, "derivative time (Td, min)":dbl}, "Abilita pid":bool, "Precisione pid W":dbl, "Medie pid":i32, "Trampa[s]":i32, "Tstab ramp[s]":i32, "Max%pid":i32}
  T48 = cluster{"proportional gain (Kc)":dbl, "integral time (Ti, min)":dbl, "derivative time (Td, min)":dbl}
  T49 = cluster{"PID gains Rpm":cluster{"proportional gain (Kc)":dbl, "integral time (Ti, min)":dbl, "derivative time (Td, min)":dbl}, "Abilita pid":bool, "Precisione pid Rpm":dbl, "Medie pid":i32, "Trampa[s]":i32, "Tstab ramp[s]":i32, "Max%pid":i32}
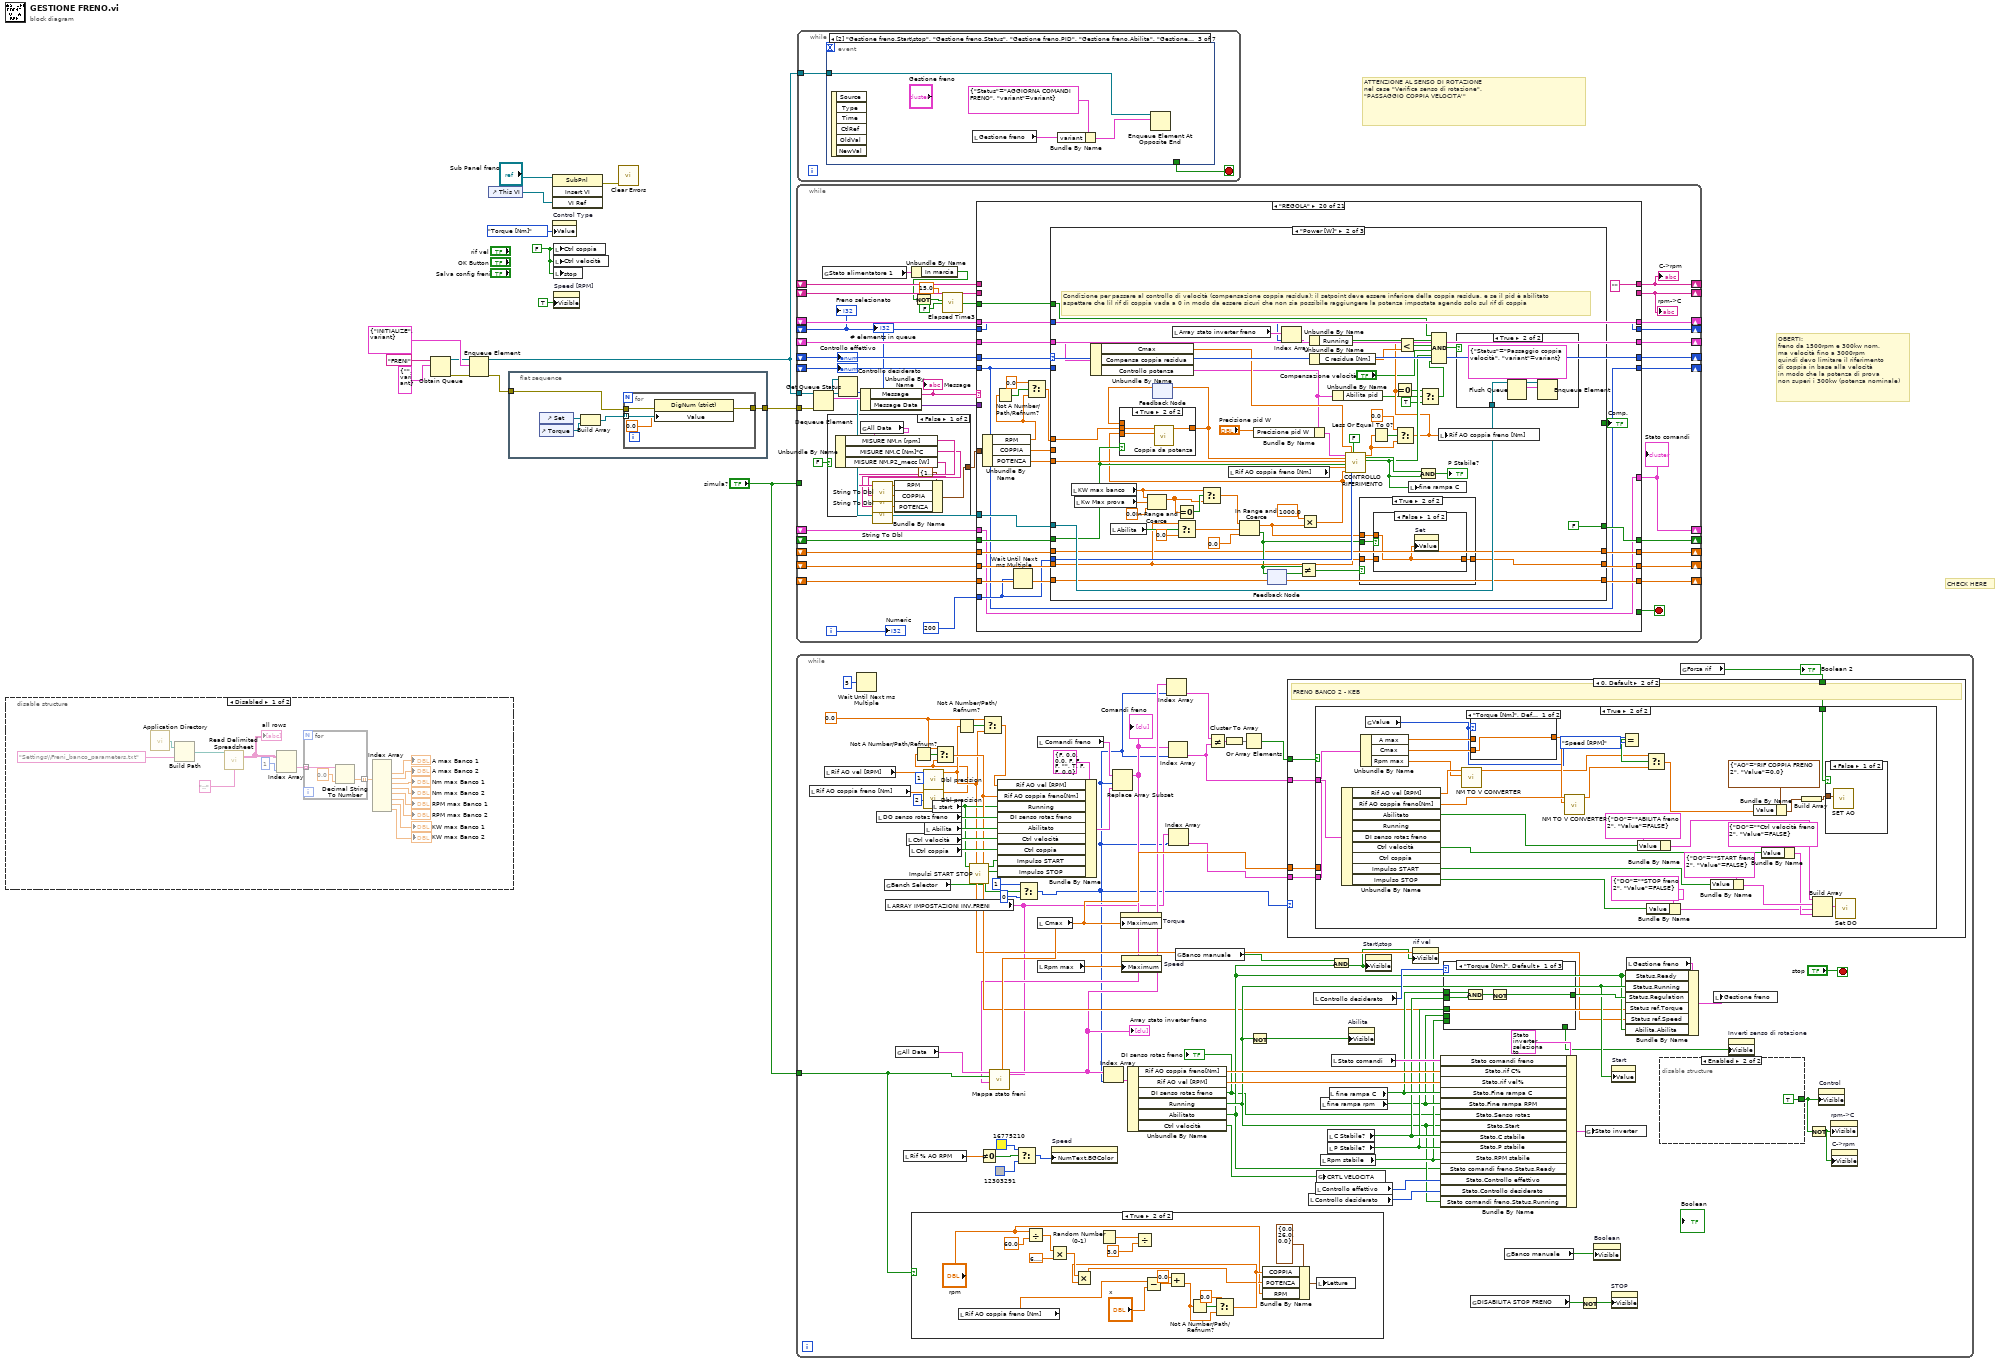
[diagram p0: block diagram]
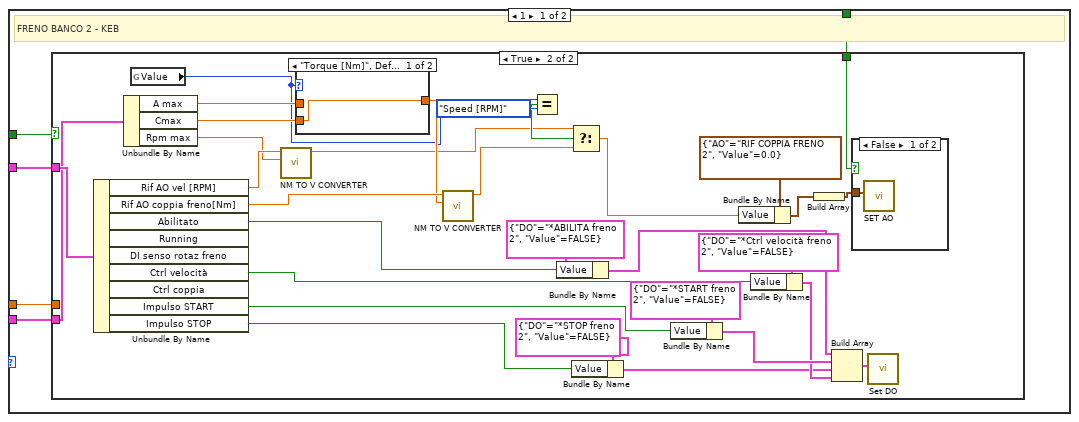
[diagram p3: hidden frame]
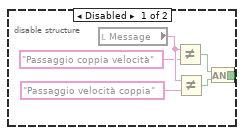
[diagram p10: hidden frame]
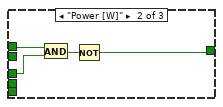
[diagram p11: hidden frame]
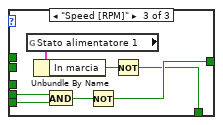
[diagram p12: hidden frame]
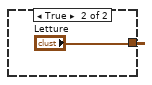
[diagram p14: hidden frame]
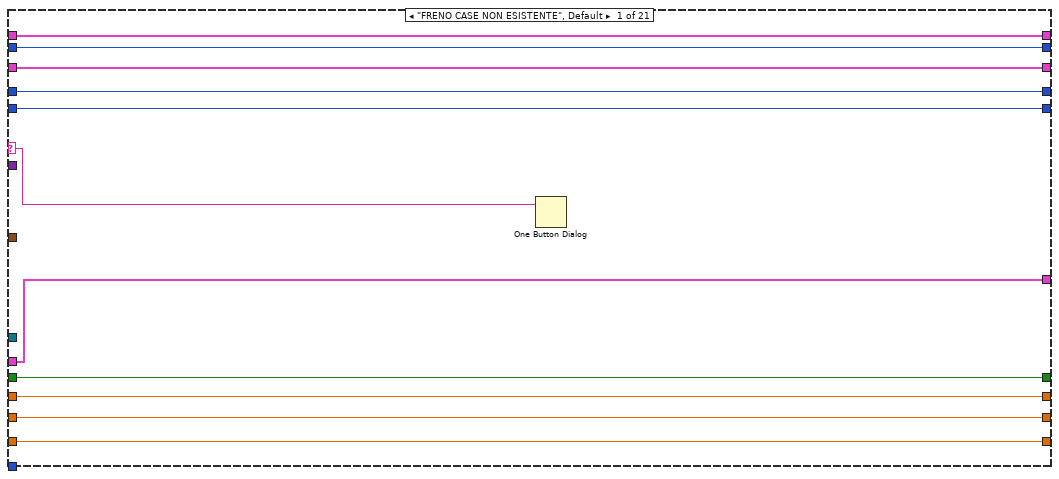
[diagram p15: hidden frame]
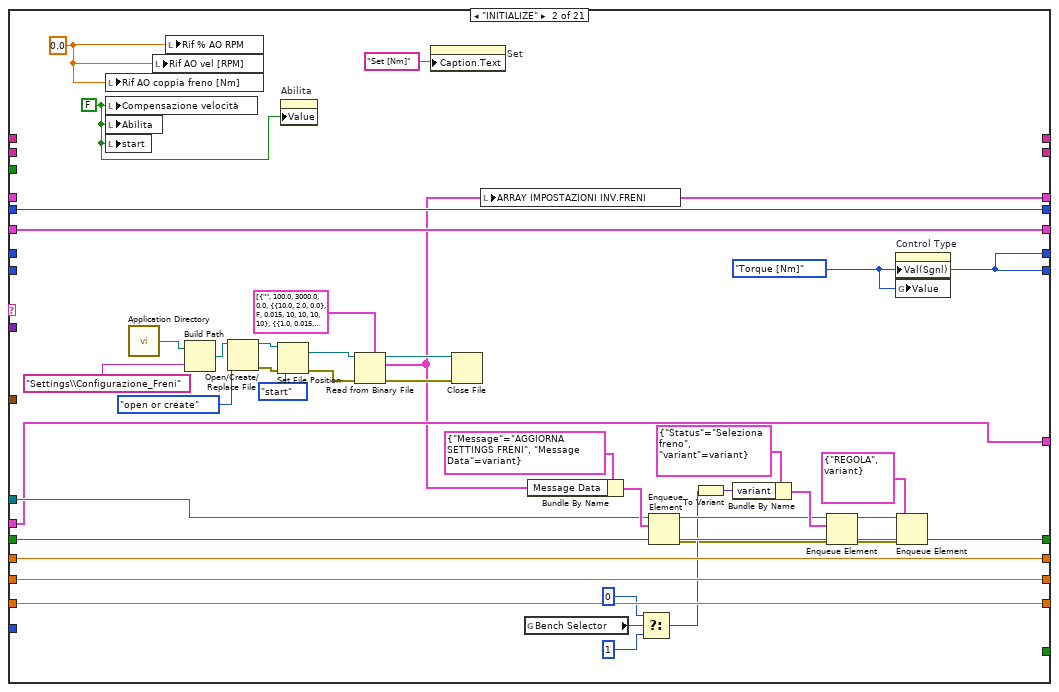
[diagram p16: hidden frame]
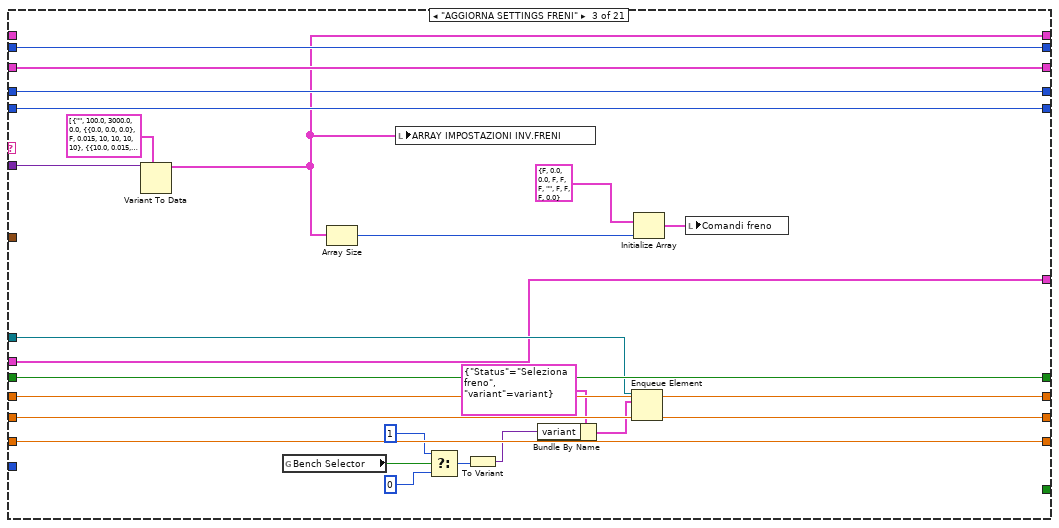
[diagram p17: hidden frame]
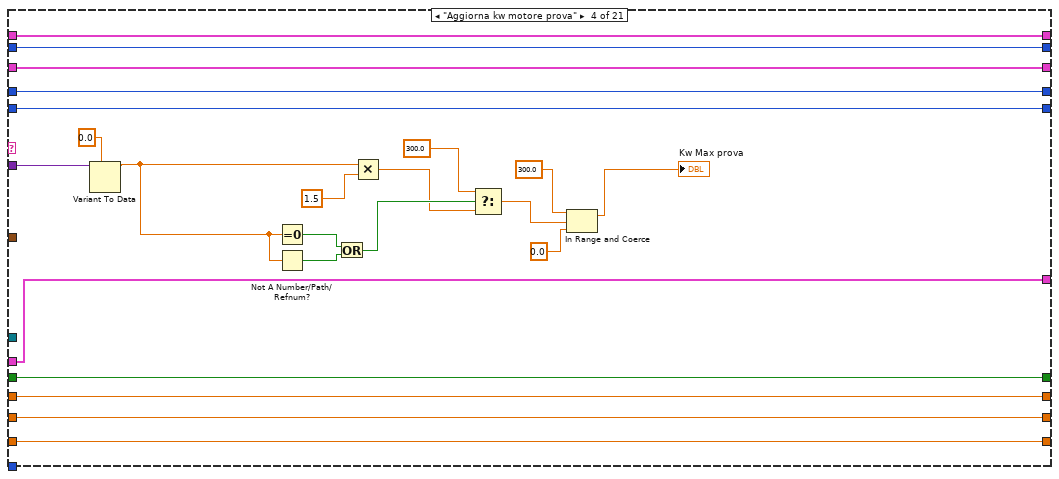
[diagram p18: hidden frame]
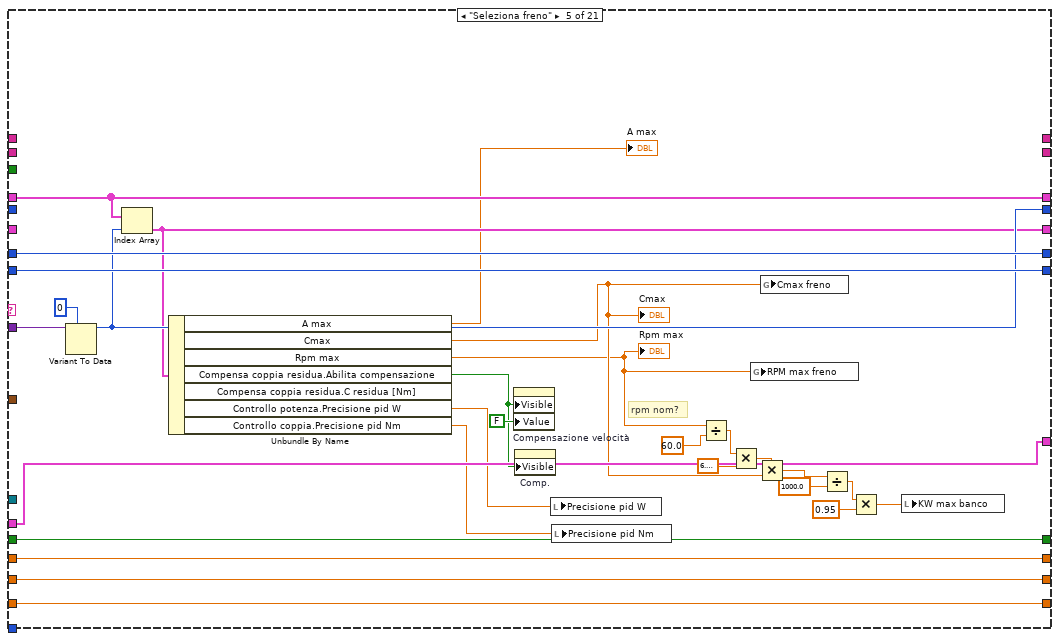
[diagram p19: hidden frame]
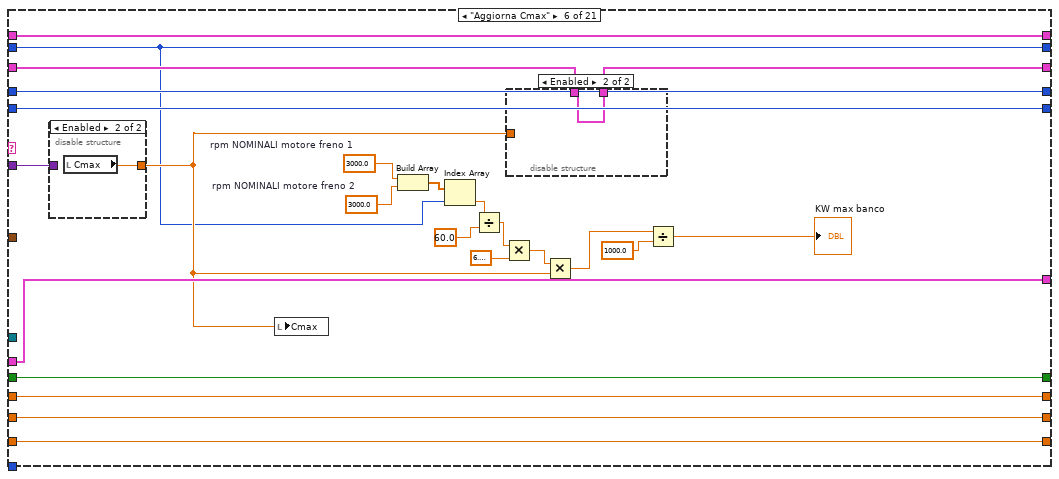
[diagram p20: hidden frame]
diagram:
  w3 = FALSE ("Ctrl coppia")
  # "CHECK HERE"
  # "ATTENZIONE AL SENSO DI ROTAZIONE \nnel case \"Verifica senso di rotazione\".  \n\"PASSAGGIO COPPIA VELOCITA'\""
  # "OBERTI:\nfreno da 1500rpm e 300kw nom. \nma velocità fino a 3000rpm\nquindi devo limitare il riferimento\ndi coppia in base alla velocità\nin modo che la potenza di prova\nnon superi i 300kw (potenza nominale)"
  n1 = disable-structure shown="Disabled" {
    frame Disabled {
      n2 = call <vilib>:"Application Directory.vi"() -> ("Application Directory"=w19:path)
      n3 = Build Path(base path=w19, name or relative path="Settings\\Freni_banco_parameters.txt") -> (appended path=w20:path)
      n4 = call-poly <vilib>:"Read Delimited Spreadsheet.vi"("file path (dialog if empty)"=w20, "delimiter (\\t)"="::" ("delimiter (\\t)")) -> ("all rows"=w21:string[][])  [unwired: 8 in, 5 out]
      "all rows" <- w21
      n5 = Index Array(array=w21, index (col)=1 ("disabled index (col)")) -> (element=w22:string[])  [unwired: 1 in]
      n6 = for {
        tunnel: w22 -> [w34] mode=indexing
        tunnel: [w33] -> w23 mode=indexing
        n7 = Decimal String To Number(string=w34, default (0L)=0.0 ("default (0 I32)")) -> (number=w33:dbl)  [unwired: 1 in, 1 out]
      }
      n8 = Index Array(array=w23) -> (element #1=→"A max Banco 1":dbl, element #2=→"A max Banco 2":dbl, element #3=→"Nm max Banco 1":dbl, element #4=→"Nm max Banco 2":dbl, element #5=→"RPM max Banco 1":dbl, element #6=→"RPM max Banco 2":dbl, element #7=→"KW max Banco 1":dbl, element #8=→"KW max Banco 2":dbl)  [unwired: 8 in]
    }
    frame Enabled {
    }
  }
  n9 = Obtain Queue(name (unnamed)="FRENI", element data type=T5 {"Message"="", "Message Data"=variant} ("Message Cluster")) -> (queue out=w12:refnum<queue>, error out=w11:errorcluster)  [unwired: 3 in, 1 out]
  n10 = Enqueue Element(queue=w12, element=cluster{"Status":string, "variant":variant} {"Status"="INITIALIZE", "variant"=variant}, error in (no error)=w11) -> (queue out=w10:refnum<queue>, error out=w2:errorcluster)  [unwired: 1 in, 1 out]
  n11 = control-ref of="This VI"() -> (w7:refnum<vi>)
  n12 = flat-sequence {
    tunnel: w2 -> [w36]
    tunnel: [w35] -> w1
    frame #0 {
      n13 = control-ref of="Set"() -> (w37:refnum<vi>)
      n14 = control-ref of="Torque"() -> (w38:refnum<vi>)
      n15 = Build Array(w37, w38) -> (w39:refnum<vi>[])
      n16 = for {
        tunnel: w39 -> [w43] mode=indexing
        tunnel: w36 -> [w41]
        tunnel: [w40] -> w35
        n17 = property class="DigNum (strict)"(reference=w43, error in=w41, "Value"=0.0) -> (error out=w40:errorcluster)  [unwired: 1 out]
      }
    }
  }
  n18 = invoke class="SubPnl" method="Insert VI"(reference="Sub Panel freno", "VI Ref"=w7) -> (error out=w6:errorcluster)  [unwired: 2 in, 3 out]
  n19 = property on="Control Type" class="RadioBtnsControl (strict)"("Value"=T2."Torque [Nm]") -> ()  [unwired: 2 in, 2 out]
  n20 = local write "Ctrl coppia"(w3) -> ()
  n21 = local write "Ctrl velocità"(w3) -> ()
  n22 = local write "stop"(w3) -> ()
  n23 = property on="Speed [RPM]" class="Bool (strict)"("Visible"=TRUE) -> ()  [unwired: 2 in, 2 out]
  n24 = call <vilib>:"Clear Errors.vi"("error in (no error)"=w6) -> ()  [unwired: 5 in, 2 out]
  n25 = while {
    tunnel: "simula?" -> [w103]
    stop <- "stop" stop-if-true
    w57 = 0.0 ("t")
    n26 = local read "Rif AO coppia freno [Nm]"() -> (w68:dbl)
    n27 = local read "Rif AO vel [RPM]"() -> (w71:dbl)
    n28 = Wait Until Next ms Multiple(millisecond multiple=u32 5) -> ()  [unwired: 1 out]
    n29 = local read "DO senso rotaz freno"() -> (w99:bool)
    n30 = global read "BenchSelector.vi" "Bench Selector"() -> (w44:bool)
    n31 = local read "ARRAY IMPOSTAZIONI INV.FRENI"() -> (w52:T4[])
    n32 = global read "Global_All_Data.vi" "All Data"() -> (w82:T11)
    n33 = local read "Rif % AO RPM"() -> (w64:dbl)
    n34 = local read "Ctrl velocità"() -> (w102:bool)
    n35 = local read "Ctrl coppia"() -> (w101:bool)
    n36 = case shown="True" w103 {
      frame False {
      }
      frame True {
        n37 = local read "Rif AO coppia freno [Nm]"() -> (w220:dbl)
        n38 = Divide(x="rpm", y=60.0) -> (x/y=w225:dbl)
        n39 = Multiply(x=w225, y=6.283185307179586) -> (x*y=w227:dbl)
        n40 = Random Number (0-1)() -> (number: 0 to 1=w230:dbl)
        n41 = Divide(x=w230, y=3.0) -> ()  [unwired: 1 out]
        n42 = Subtract(x=w220, y="x") -> (x-y=w235:dbl)
        n43 = Add(x=0.0, y=w235) -> (x+y=w232:dbl)
        n44 = Not A Number/Path/Refnum?(number/path/refnum=w232) -> (NaN/Path/Refnum?=w233:bool)
        n45 = Select(t=0.0, s=w233, f=w232) -> (s? t:f=w223:dbl)
        n46 = Multiply(x=w227, y=w223) -> (x*y=w222:dbl)
        n47 = Bundle By Name(cluster=cluster{"RPM":dbl, "COPPIA":dbl, "POTENZA":dbl} {"RPM"=0.0, "COPPIA"=26.0, "POTENZA"=0.0} ("Letture"), "COPPIA"=w223, "POTENZA"=w222, "RPM"="rpm") -> (w236:cluster{"RPM":dbl, "COPPIA":dbl, "POTENZA":dbl})
        n48 = local write "Letture"(w236) -> ()
      }
    }
    n49 = call "Dbl precision.vi"("precision (6)"=i16 1, "Numeric in"=w71) -> ("Numeric out"=w70:dbl)  [unwired: 9 in]
    n50 = call "Dbl precision.vi"("precision (6)"=i16 2, "Numeric in"=w68) -> ("Numeric out"=w67:dbl)  [unwired: 9 in]
    n51 = Not A Number/Path/Refnum?(number/path/refnum=w67) -> (NaN/Path/Refnum?=w77:bool)
    n52 = local read "Abilita"() -> (w108:bool)
    n53 = local read "start"() -> (w72:bool)
    n54 = Select(t=w57, s=w77, f=w67) -> (s? t:f=w76:dbl)
    n55 = Not A Number/Path/Refnum?(number/path/refnum=w70) -> (NaN/Path/Refnum?=w79:bool)
    n56 = call "Impulsi START STOP.vi"("Segnale"=w72) -> ("STOP"=w73:bool, "START"=w74:bool)  [unwired: 9 in]
    n57 = Not Equal To 0?(x=w64) -> (x != 0?=w63:bool)
    n58 = Select(t=w57, s=w79, f=w70) -> (s? t:f=w78:dbl)
    n59 = Bundle By Name(cluster=T1 {"DI senso rotaz freno"=FALSE, "Rif AO vel [RPM]"=0.0, "Rif AO coppia freno[Nm]"=0.0, "Abilitato"=FALSE, "Running"=FALSE, "Ctrl velocità"=FALSE, "Nome"="", "Ctrl coppia"=TRUE, "Impulso START"=FALSE, "Impulso STOP"=FALSE, "Rif AO Corr [A] "=0.0} ("Stato inverter"), "Rif AO vel [RPM]"=w78, "Rif AO coppia freno[Nm]"=w76, "Running"=w72, "DI senso rotaz freno"=w99, "Abilitato"=w108, "Ctrl velocità"=w102, "Ctrl coppia"=w101, "Impulso START"=w74, "Impulso STOP"=w73) -> (w119:T1)
    n60 = Select(t=u32 16775210 ("Numeric Text.Text Colors:BG Color"), s=w63, f=u32 12303291 ("Numeric Text.Text Colors:BG Color")) -> (s? t:f=w61:u32)
    n61 = Select(t=1 ("Freno selezionato"), s=w44, f=0 ("Freno selezionato")) -> (s? t:f=w47:i32)
    n62 = local read "Rpm max"() -> (w104:dbl)
    n63 = local read "Comandi freno"() -> (w111:T1[])
    n64 = local read "Cmax"() -> (w86:dbl)
    n65 = property on="Speed" class="DigNum (strict)"("NumText.BGColor"=w61) -> ()  [unwired: 2 in, 2 out]
    n66 = Replace Array Subset(array=w111, new element=w119, index=w47) -> (w54:T1[])
    "Comandi freno" <- w54
    n67 = call "Mappa stato freni.vi"("Cmax"=w86, "ARRAY IMPOSTAZIONI INV.FRENI"=w52, "Array"=w54, "simula?"=w103, "All Data"=w82) -> ("Array stato freni"=w56:T1[])  [unwired: 6 in]
    "Array stato inverter freno" <- w56
    n68 = Index Array(array=w56, index=w47) -> (element=w116:T1)
    n69 = property on="Torque" class="DigNum (strict)"("Maximum"=w86) -> ()  [unwired: 2 in, 2 out]
    n70 = property on="Speed" class="DigNum (strict)"("Maximum"=w104) -> ()  [unwired: 2 in, 2 out]
    n71 = Unbundle By Name(w116) -> ("Rif AO coppia freno[Nm]"=w107:dbl, "Rif AO vel [RPM]"=w106:dbl, "DI senso rotaz freno"=w58:bool, "Running"=w85:bool, "Abilitato"=w83:bool, "Ctrl velocità"=w100:bool)
    "DI senso rotaz freno" <- w58
    n72 = Index Array(array=w56, index=w47) -> (element=w55:T1)
    n73 = Index Array(array=w54, index=w47) -> (element=w53:T1)
    n74 = Index Array(array=w52, index=w47) -> (element=w51:T4)
    n75 = global read "Global FINE AVVIO.vi" "Banco manuale"() -> (w75:bool)
    n76 = Not Equal?(x=w55, y=w53) -> (x != y?=w50:T38)
    n77 = Cluster To Array(cluster=w50) -> (array=w49:bool[])
    n78 = Or Array Elements(Boolean array=w49) -> (logical OR=w48:bool)
    n79 = Not(x=w85) -> (.not. x?=w105:bool)
    n80 = local read "Controllo desiderato"() -> (w90:T2)
    n81 = local read "Controllo desiderato"() -> (w98:T2)
    n82 = local read "Controllo effettivo"() -> (w91:T2)
    n83 = global write "Global CTRL VELOCITA.vi" "CRTL VELOCITA"(w100) -> ()
    n84 = local read "fine rampa rpm"() -> (w93:bool)
    n85 = local read "Rpm stabile"() -> (w92:bool)
    n86 = local read "C Stabile?"() -> (w96:bool)
    n87 = local read "P Stabile?"() -> (w94:bool)
    n88 = local read "fine rampa C"() -> (w97:bool)
    n89 = And(x=w75, y=w83) -> (x .and. y?=w59:bool)
    n90 = local read "Stato comandi"() -> (w114:T3)
    n91 = property on="Abilita" class="Clust (strict)"("Visible"=w105) -> ()  [unwired: 2 in, 2 out]
    n92 = property on="Start\\stop" class="Clust (strict)"("Visible"=w59) -> ()  [unwired: 2 in, 2 out]
    n93 = property on="rif vel" class="Bool"("Visible"=w59) -> ()  [unwired: 2 in, 2 out]
    n94 = Bundle By Name(cluster=T6 {"Stato comandi freno"={"Control"={"Control Type"=enum."Torque [Nm]", "Set"=0.0, "Inverti senso di rotazione"=FALSE}, "Start\\stop"={"Start"=FALSE, "STOP"=FALSE}, "Status"={"Ready"=FALSE, "Running"=FALSE, "Regulation"=FALSE}, "PID"=FALSE, "Abilita"={"Abilita"=FALSE}, "Status ref"={"Torque"=0.0, "Speed"=0.0}}, "Stato"={"rif C%"=0.0, "rif vel%"=0.0, "Controllo effettivo"=enum."Torque [Nm]", "Controllo desiderato"=enum."Torque [Nm]", "Fine rampa C"=FALSE, "Fine rampa RPM"=FALSE, "Senso rotaz"=FALSE, "Start"=FALSE, "C stabile"=FALSE, "P stabile"=FALSE, "RPM stabile"=FALSE}} ("Stato inverter"), "Stato comandi freno"=w114, "Stato.rif C%"=w107, "Stato.rif vel%"=w106, "Stato.Fine rampa C"=w97, "Stato.Fine rampa RPM"=w93, "Stato.Senso rotaz"=w58, "Stato.Start"=w85, "Stato.C stabile"=w96, "Stato.P stabile"=w94, "Stato.RPM stabile"=w92, "Stato comandi freno.Status.Ready"=w83, "Stato.Controllo effettivo"=w91, "Stato.Controllo desiderato"=w90, "Stato comandi freno.Status.Running"=w85) -> (w113:T6)
    n95 = case shown="\"Torque [Nm]\", Default" w98 {
      tunnel: w97 -> [w207 w212 _]
      tunnel: w96 -> [w208 _ _]
      tunnel: [w205 w209 w216] -> w95
      tunnel: w94 -> [_ w211 _]
      tunnel: w93 -> [_ _ w219]
      tunnel: w92 -> [_ _ w218]
      tunnel: [_ _ w213] -> w84
      frame "Torque [Nm]", Default {
        n96 = And(x=w207, y=w208) -> (x .and. y?=w206:bool)
        n97 = Not(x=w206) -> (.not. x?=w205:bool)
      }
      frame "Power [W]" {
        n98 = And(x=w212, y=w211) -> (x .and. y?=w210:bool)
        n99 = Not(x=w210) -> (.not. x?=w209:bool)
      }
      frame "Speed [RPM]" {
        n100 = global read "Stato alimentatore 1.vi" "Stato alimentatore 1"() -> (w215:T40)
        n101 = Unbundle By Name(w215) -> ("In marcia"=w214:bool)
        n102 = And(x=w219, y=w218) -> (x .and. y?=w217:bool)
        n103 = Not(x=w217) -> (.not. x?=w216:bool)
        n104 = Not(x=w214) -> (.not. x?=w213:bool)
      }
    }
    n105 = global read "Fine rampa sinus penta.vi" "DISABILITA STOP FRENO"() -> (w81:bool)
    n106 = global read "Global FINE AVVIO.vi" "Banco manuale"() -> (w89:bool)
    n107 = Not(x=w81) -> (.not. x?=w80:bool)
    n108 = global write "Stato comandi freno.vi" "Stato inverter"(w113) -> ()
    n109 = property on="Boolean" class="Bool (strict)"("Visible"=w89) -> ()  [unwired: 2 in, 2 out]
    n110 = property on="STOP" class="Bool (strict)"("Visible"=w80) -> ()  [unwired: 2 in, 2 out]
    n111 = property on="Start" class="Bool (strict)"("Value"=w85) -> ()  [unwired: 2 in, 2 out]
    n112 = local read "Gestione freno"() -> (w110:T3)
    n113 = Bundle By Name(cluster=w110, "Status.Ready"=w83, "Status.Running"=w85, "Status.Regulation"=w95, "Status ref.Torque"=w76, "Status ref.Speed"=w70, "Abilita.Abilita"=w83) -> (w109:T3)
    n114 = disable-structure shown="Enabled" {
      disable-tunnel: [w198 TRUE] -> w88
      frame Disabled {
        n115 = local read "Message"() -> (w201:string)
        n116 = Not Equal?(x=w201, y="Passaggio coppia velocità") -> (x != y?=w200:bool)
        n117 = Not Equal?(x=w201, y="Passaggio velocità coppia") -> (x != y?=w202:bool)
        n118 = And(x=w200, y=w202) -> (x .and. y?=w198:bool)
      }
      frame Enabled {
      }
    }
    n119 = global read "Global Trampa 0.vi" "Forza rif"() -> (w65:bool)
    "Boolean 2" <- w65
    n120 = case shown="0, Default" w47 {
      tunnel: w53 -> [w124 w163]
      tunnel: w48 -> [w123 w162]
      tunnel: w51 -> [w122 w161]
      tunnel: w86 -> [w121 w160]
      tunnel: w65 -> [w120 w159]
      frame 1 {
        # "FRENO BANCO 2 - KEB"
        n121 = case shown="True" w123 {
          tunnel: w124 -> [_ w155]
          tunnel: w122 -> [_ w147]
          tunnel: w121 -> [_ _]
          tunnel: w120 -> [_ w137]
          frame False {
          }
          frame True {
            n122 = Unbundle By Name(w155) -> ("Rif AO vel [RPM]"=w135:dbl, "Rif AO coppia freno[Nm]"=w136:dbl, "Abilitato"=w145:bool, "Ctrl velocità"=w146:bool, "Impulso START"=w143:bool, "Impulso STOP"=w139:bool)  [unwired: 3 out]
            n123 = Unbundle By Name(w147) -> ("A max"=w132:dbl, "Cmax"=w131:dbl, "Rpm max"=w133:dbl)
            n124 = global read "Global control type freno.vi" "Value"() -> (w130:T2)
            n125 = call "NM TO V CONVERTER.vi"("Max Banco"=w133, "Set Point"=w135) -> ("Set Value to cDAQ"=w125:dbl)  [unwired: 8 in, 1 out]
            n126 = case shown="\"Torque [Nm]\", Default" w130 {
              tunnel: [w156 w157] -> w134
              tunnel: w132 -> [_ w157]
              tunnel: w131 -> [w156 _]
              frame "Torque [Nm]", Default {
              }
              frame "Corrente [A]" {
              }
            }
            n127 = call "NM TO V CONVERTER.vi"("Max Banco"=w134, "Set Point"=w136) -> ("Set Value to cDAQ"=w127:dbl)  [unwired: 8 in, 1 out]
            n128 = Equal?(x=w130, y=T2."Speed [RPM]") -> (x = y?=w128:bool)
            n129 = Bundle By Name(cluster=T7 {"DO"=enum."*ABILITA freno 2", "Value"=FALSE} ("Cluster SET DO"), "Value"=w145) -> (w142:T7)
            n130 = Select(t=w125, s=w128, f=w127) -> (s? t:f=w126:dbl)
            n131 = Bundle By Name(cluster=T7 {"DO"=enum."*STOP freno 2", "Value"=FALSE} ("Cluster SET DO"), "Value"=w139) -> (w140:T7)
            n132 = Bundle By Name(cluster=T7 {"DO"=enum."*START freno 2", "Value"=FALSE} ("Cluster SET DO"), "Value"=w143) -> (w149:T7)
            n133 = Bundle By Name(cluster=T9 {"AO"=enum."RIF COPPIA FRENO 2", "Value"=0.0} ("Cluster SET AO"), "Value"=w126) -> (w152:T9)
            n134 = Bundle By Name(cluster=T7 {"DO"=enum."*Ctrl velocità freno 2", "Value"=FALSE} ("Cluster SET DO"), "Value"=w146) -> (w141:T7)
            n135 = Build Array(w152) -> (w154:T9[])
            n136 = Build Array(w142, w149, w140, w141) -> (w148:T7[])
            n137 = case shown="False" w137 {
              tunnel: w154 -> [w158 _]
              frame False {
                n138 = call "SET AO.vi"("Cluster SET AO"=w158) -> ()  [unwired: 10 in, 1 out]
              }
              frame True {
              }
            }
            n139 = call "Set DO.vi"("Cluster SET DO"=w148) -> ()  [unwired: 10 in, 1 out]
          }
        }
      }
      frame 0, Default {
        # "FRENO BANCO 2 - KEB"
        n140 = case shown="True" w162 {
          tunnel: w163 -> [_ w194]
          tunnel: w161 -> [_ w186]
          tunnel: w160 -> [_ _]
          tunnel: w159 -> [_ w176]
          frame False {
          }
          frame True {
            n141 = Unbundle By Name(w194) -> ("Rif AO vel [RPM]"=w174:dbl, "Rif AO coppia freno[Nm]"=w175:dbl, "Abilitato"=w184:bool, "Ctrl velocità"=w185:bool, "Impulso START"=w182:bool, "Impulso STOP"=w178:bool)  [unwired: 3 out]
            n142 = Unbundle By Name(w186) -> ("A max"=w171:dbl, "Cmax"=w170:dbl, "Rpm max"=w172:dbl)
            n143 = global read "Global control type freno.vi" "Value"() -> (w169:T2)
            n144 = call "NM TO V CONVERTER.vi"("Max Banco"=w172, "Set Point"=w174) -> ("Set Value to cDAQ"=w164:dbl)  [unwired: 8 in, 1 out]
            n145 = case shown="\"Torque [Nm]\", Default" w169 {
              tunnel: [w195 w196] -> w173
              tunnel: w171 -> [_ w196]
              tunnel: w170 -> [w195 _]
              frame "Torque [Nm]", Default {
              }
              frame "Corrente [A]" {
              }
            }
            n146 = call "NM TO V CONVERTER.vi"("Max Banco"=w173, "Set Point"=w175) -> ("Set Value to cDAQ"=w166:dbl)  [unwired: 8 in, 1 out]
            n147 = Equal?(x=w169, y=T2."Speed [RPM]") -> (x = y?=w167:bool)
            n148 = Bundle By Name(cluster=T7 {"DO"=enum."*ABILITA freno 2", "Value"=FALSE} ("Cluster SET DO"), "Value"=w184) -> (w181:T7)
            n149 = Select(t=w164, s=w167, f=w166) -> (s? t:f=w165:dbl)
            n150 = Bundle By Name(cluster=T7 {"DO"=enum."*STOP freno 2", "Value"=FALSE} ("Cluster SET DO"), "Value"=w178) -> (w179:T7)
            n151 = Bundle By Name(cluster=T7 {"DO"=enum."*START freno 2", "Value"=FALSE} ("Cluster SET DO"), "Value"=w182) -> (w188:T7)
            n152 = Bundle By Name(cluster=T9 {"AO"=enum."RIF COPPIA FRENO 2", "Value"=0.0} ("Cluster SET AO"), "Value"=w165) -> (w191:T9)
            n153 = Bundle By Name(cluster=T7 {"DO"=enum."*Ctrl velocità freno 2", "Value"=FALSE} ("Cluster SET DO"), "Value"=w185) -> (w180:T7)
            n154 = Build Array(w191) -> (w193:T9[])
            n155 = Build Array(w181, w188, w179, w180) -> (w187:T7[])
            n156 = case shown="False" w176 {
              tunnel: w193 -> [w197 _]
              frame False {
                n157 = call "SET AO.vi"("Cluster SET AO"=w197) -> ()  [unwired: 10 in, 1 out]
              }
              frame True {
              }
            }
            n158 = call "Set DO.vi"("Cluster SET DO"=w187) -> ()  [unwired: 10 in, 1 out]
          }
        }
      }
    }
    n159 = local write "Gestione freno"(w109) -> ()
    n160 = property on="Inverti senso di rotazione" class="Bool (strict)"("Visible"=w84) -> ()  [unwired: 2 in, 2 out]
    n161 = Not(x=w88) -> (.not. x?=w87:bool)
    n162 = property on="Control" class="Clust (strict)"("Visible"=w88) -> ()  [unwired: 2 in, 2 out]
    n163 = property on="rpm->C" class="Str"("Visible"=w87) -> ()  [unwired: 2 in, 2 out]
    n164 = property on="C->rpm" class="Str"("Visible"=w87) -> ()  [unwired: 2 in, 2 out]
  }
  n165 = while {
    tunnel: w10 -> [w279]
    tunnel: w1 -> [w278]
    shift-right: [w273] -> _
    shift-left: _ -> [w274]
    shift-right: [w272] -> _
    shift-left: _ -> [w271]
    shift-right: [w270] -> _
    shift-left: _ -> [w269]
    shift-right: [w268] -> _
    shift-left: _ -> [w267]
    shift-right: [w266] -> _
    shift-left: _ -> [w265]
    shift-right: [w264] -> _
    shift-left: _ -> [w263]
    shift-right: [w261] -> _
    shift-left: _ -> [w262]
    shift-right: [w247] -> _
    shift-left: _ -> [w258]
    shift-right: [w257] -> _
    shift-left: _ -> [w256]
    shift-right: [w254] -> _
    shift-left: _ -> [w253]
    shift-right: [w252] -> _
    shift-left: _ -> [w251]
    shift-right: [w249] -> _
    shift-left: _ -> [w250]
    tunnel: "simula?" -> [_]
    i -> [w255]
    stop <- w259 stop-if-true
    n166 = Dequeue Element(queue=w279, error in (no error)=w278) -> (queue out=w239:refnum<queue>, element=w277:T5)  [unwired: 1 in, 2 out]
    n167 = global read "Stato alimentatore 1.vi" "Stato alimentatore 1"() -> (w245:T40)
    n168 = case shown="False" FALSE {
      tunnel: [w280 "Letture"] -> w248
      frame False {
        n169 = global read "Global_All_Data.vi" "All Data"() -> (w288:T11)
        n170 = Unbundle By Name(w288) -> ("MISURE NM.n [rpm]"=w287:string, "MISURE NM.C [Nm]*C"=w286:string, "MISURE NM.P2_mecc [W]"=w285:string)
        n171 = call "String To Dbl.vi"("String"=w287) -> ("Numeric"=w283:dbl)  [unwired: 10 in]
        n172 = call "String To Dbl.vi"("String"=w286) -> ("Numeric"=w282:dbl)  [unwired: 10 in]
        n173 = call "String To Dbl.vi"("String"=w285) -> ("Numeric"=w281:dbl)  [unwired: 10 in]
        n174 = Bundle By Name(cluster=cluster{"RPM":dbl, "COPPIA":dbl, "POTENZA":dbl} {"RPM"=1170.0, "COPPIA"=50.475222156442, "POTENZA"=6184.330897484647} ("Letture"), "RPM"=w283, "COPPIA"=w282, "POTENZA"=w281) -> (w280:cluster{"RPM":dbl, "COPPIA":dbl, "POTENZA":dbl})
      }
      frame True {
      }
    }
    n175 = Get Queue Status(queue=w239) -> (# elements in queue=→"# elements in queue":i32)  [unwired: 2 in, 7 out]
    n176 = Unbundle By Name(w277) -> ("Message"=w276:string, "Message Data"=w275:variant)
    "Message" <- w276
    n177 = Unbundle By Name(w245) -> ("In marcia"=w241:bool)
    n178 = Not(x=w241) -> (.not. x?=w244:bool)
    n179 = call "Elapsed Time3"("Time Target (s)"=15.0, "Reset"=w244, "Auto Reset"=FALSE) -> ("Time has Elapsed"=w240:bool)  [unwired: 9 in, 7 out]
    n180 = case shown="\"REGOLA\"" w276 {
      selector: w276 -> [w290 _ _ _ _ _ _ _ _ _ _ _ _ _ _ _ _ _ _ _ _]
      tunnel: w275 -> [_ _ w354 w375 w413 w428 w455 w469 w481 w505 _ _ _ _ _ w668 w691 _ _ _ _]
      tunnel: w274 -> [w300 _ _ w385 w411 w437 w457 w472 w484 w509 w570 w581 w591 w609 w632 w670 w701 w704 w974 w1187 w1458]
      tunnel: [w300 w317 w345 w385 w411 w437 w457 w472 w484 w509 w570 w581 w591 w609 w632 w670 w701 w704 w974 w1187 w1458] -> w273
      tunnel: [w299 w339 w362 w384 w402 w429 w456 w471 w483 w501 w569 w580 w590 w608 w631 w669 w700 w718 w958 w1198 w1457] -> w272
      tunnel: w271 -> [w299 w339 w362 w384 _ w419 w456 w471 w483 w502 w569 w580 w590 w608 w631 w669 w700 w718 w958 w1198 w1457]
      tunnel: w248 -> [_ _ _ _ _ _ _ _ _ _ _ _ _ _ _ w656 _ w719 w972 w1199 _]
      tunnel: [w298 w315 w361 w383 w407 w436 w453 w466 w478 w508 w568 w579 w586 w601 w627 w663 w699 w716 w966 w1197 w1456] -> w270
      tunnel: w269 -> [w298 _ w361 w383 w407 w436 w453 w466 w478 w508 w568 w579 w586 w601 w627 w664 w699 w717 w967 w1197 w1456]
      tunnel: [w297 w338 w360 w382 w410 w435 w448 w468 w480 w497 w567 w578 w589 w607 w630 w653 w698 w712 w973 w1194 w1455] -> w268
      tunnel: w267 -> [w297 w338 w360 w382 w410 w435 _ w468 w480 w497 w567 w578 w589 w607 w630 _ w698 w712 w973 w1195 w1455]
      tunnel: [w296 w315 w359 w381 w406 w434 w452 w465 w477 w500 w566 w577 w585 w604 w626 w638 w697 w715 w968 w1180 w1454] -> w266
      tunnel: w265 -> [w296 _ w359 w381 w406 w434 w452 w465 w477 w500 w566 w577 w585 w604 w626 _ w697 w715 w968 w1180 w1454]
      tunnel: w239 -> [_ w327 w350 _ _ _ _ _ _ w496 _ _ _ w600 _ w649 _ w714 w965 w1190 _]
      tunnel: [w295 w337 w358 w380 w409 w433 w447 w460 w479 w498 w565 w576 w588 w606 w629 w646 w696 w711 w970 w1191 w1453] -> w264
      tunnel: w263 -> [w295 w337 w358 w380 w409 w433 w447 _ w479 w498 w565 w576 w588 w606 w629 _ w696 w711 w970 w1192 w1453]
      tunnel: w262 -> [w294 w336 w357 w379 w408 w432 w446 w467 _ w499 w564 w575 w587 w605 w628 _ w695 _ w975 w1189 w1452]
      tunnel: [w294 w336 w357 w379 w408 w432 w446 w467 w473 w499 w564 w575 w587 w605 w628 w650 w695 w702 w975 w1188 w1452] -> w261
      tunnel: u32 200 ("millisecond multiple") -> [_ _ _ _ _ _ _ _ _ _ _ _ _ _ _ _ _ w707 w960 w1183 _]
      tunnel: [_ _ _ _ _ _ _ _ _ _ _ _ _ _ _ _ _ _ _ _ TRUE] -> w259
      tunnel: [_ _ _ _ _ _ _ _ _ _ _ _ _ _ _ _ _ w710 _ "" _] -> w247
      tunnel: w258 -> [_ _ _ _ _ _ _ _ _ _ _ _ _ _ _ _ _ w705 _ _ _]
      tunnel: [_ _ _ _ _ _ _ _ _ _ _ _ _ _ _ _ _ _ w963 _ _] -> w257
      tunnel: w256 -> [_ _ _ _ _ _ _ _ _ _ _ _ _ _ _ _ _ _ w962 _ _]
      tunnel: [w293 w334 w356 w378 w405 w415 w451 w464 w476 w507 w563 w574 w584 w597 w625 w665 w694 w709 w961 w1181 w1450] -> w254
      tunnel: w253 -> [w293 w334 w356 w378 _ w415 w451 w464 w476 w507 w563 w574 w584 w597 w625 w665 w694 w709 w961 w1181 w1450]
      tunnel: [w292 w333 w355 w377 w404 w431 TRUE TRUE TRUE w506 w562 w573 w583 w603 w624 TRUE w693 w708 w957 w1184 w1449] -> w252
      tunnel: w251 -> [w292 w333 w355 w377 w404 w431 _ _ _ w506 w562 w573 w583 w603 w624 _ w693 w708 w957 w1185 w1449]
      tunnel: [w291 w325 w349 w376 w403 w430 w449 w462 w474 w494 w561 w572 w582 w602 w623 w654 w692 w706 w959 w1182 w1448] -> w249
      tunnel: w250 -> [w291 w325 w349 w376 w403 w430 w449 w462 w474 _ w561 w572 w582 w602 w623 w654 w692 w706 w959 w1182 w1448]
      tunnel: w240 -> [_ _ _ _ _ _ _ _ _ _ _ _ _ _ _ _ _ _ _ w1178 _]
      frame "FRENO CASE NON ESISTENTE", Default {
        n181 = One Button Dialog(message=w290) -> ()  [unwired: 1 in, 1 out]
      }
      frame "INITIALIZE" {
        w315 = T2."Torque [Nm]" ("Value")
        w303 = FALSE ("Compensazione velocità")
        w304 = 0.0 ("Stato %Rif AO coppia freno")
        n182 = local write "Rif AO coppia freno [Nm]"(w304) -> ()
        n183 = local write "Compensazione velocità"(w303) -> ()
        n184 = local write "Abilita"(w303) -> ()
        n185 = local write "start"(w303) -> ()
        n186 = call <vilib>:"Application Directory.vi"() -> ("Application Directory"=w319:path)
        n187 = local write "Rif AO vel [RPM]"(w304) -> ()
        n188 = local write "Rif % AO RPM"(w304) -> ()
        n189 = Build Path(base path=w319, name or relative path="Settings\\Configurazione_Freni") -> (appended path=w324:path)
        n190 = Open/Create/Replace File(file path (use dialog)=w324, operation (0:open)=T41."open or create") -> (refnum out=w314:refnum<file>, error out=w313:errorcluster)  [unwired: 4 in, 1 out]
        n191 = Set File Position(refnum=w314, from (0:start)=enum16{"start", "end", "current"}."start", error in=w313) -> (refnum out=w312:refnum<file>, error out=w311:errorcluster)  [unwired: 1 in]
        n192 = property on="Abilita" class="Bool (strict)"("Value"=w303) -> ()  [unwired: 2 in, 2 out]
        n193 = Read from Binary File(5:T4[] [{"Nome"="", "Cmax"=100.0, "Rpm max"=3000.0, "A max"=0.0, "Controllo RPM"={"PID gains Rpm"={"proportional gain (Kc)"=10.0, "integral time (Ti, min)"=2.0, "derivative time (Td, min)"=0.0}, "Abilita pid"=FALSE, "Precisione pid Rpm"=0.015, "Medie pid"=10, "Trampa[s]"=10, "Tstab ramp[s]"=10, "Max%pid"=10}, "Controllo coppia"={"PID gains Coppia"={"proportional gain (Kc)"=1.0, "integral time (Ti, min)"=0.015, "derivative time (Td, min)"=0.0}, "Abilita pid"=TRUE, "Precisione pid Nm"=1.0, "Medie pid"=10, "Trampa[s]"=10, "Tstab ramp[s]"=10, "Max%pid"=10}, "Controllo potenza"={"PID gains potenza"={"proportional gain (Kc)"=0.004, "integral time (Ti, min)"=0.025, "derivative time (Td, min)"=0.0}, "Abilita pid"=TRUE, "Precisione pid W"=1.0, "Medie pid"=10, "Trampa[s]"=10, "Tstab ramp[s]"=10, "Max%pid"=10}, "Compensa coppia residua"={"Abilita compensazione"=FALSE, "C residua [Nm]"=0.0, "C isteresi [Nm]"=0.0, "PID gains C-RPM"={"proportional gain (Kc)"=1.0, "integral time (Ti, min)"=0.01, "derivative time (Td, min)"=0.0}, "C precision [Nm]"=0.0, "Max%pid"=0, "Medie pid"=0}}, {"Nome"="", "Cmax"=200.0, "Rpm max"=4500.0, "A max"=0.0, "Controllo RPM"={"PID gains Rpm"={"proportional gain (Kc)"=10.0, "integral time (Ti, min)"=2.0, "derivative time (Td, min)"=0.0}, "Abilita pid"=FALSE, "Precisione pid Rpm"=0.015, "Medie pid"=10, "Trampa[s]"=10, "Tstab ramp[s]"=10, "Max%pid"=10}, "Controllo coppia"={"PID gains Coppia"={"proportional gain (Kc)"=1.0, "integral time (Ti, min)"=0.015, "derivative time (Td, min)"=0.0}, "Abilita pid"=FALSE, "Precisione pid Nm"=0.0, "Medie pid"=0, "Trampa[s]"=10, "Tstab ramp[s]"=10, "Max%pid"=10}, "Controllo potenza"={"PID gains potenza"={"proportional gain (Kc)"=0.004, "integral time (Ti, min)"=0.025, "derivative time (Td, min)"=0.0}, "Abilita pid"=FALSE, "Precisione pid W"=1.0, "Medie pid"=10, "Trampa[s]"=10, "Tstab ramp[s]"=10, "Max%pid"=10}, "Compensa coppia residua"={"Abilita compensazione"=FALSE, "C residua [Nm]"=0.0, "C isteresi [Nm]"=0.0, "PID gains C-RPM"={"proportional gain (Kc)"=1.0, "integral time (Ti, min)"=0.01, "derivative time (Td, min)"=0.0}, "C precision [Nm]"=0.0, "Max%pid"=0, "Medie pid"=0}}] ("ARRAY IMPOSTAZIONI INV.FRENI"), 8:w311, 11:w312) -> (0:w321:errorcluster, 2:w317:T4[], 3:w322:refnum<file>)  [unwired: 3 in, 1 out]
        n194 = property on="Set" class="DigNum (strict)"("Caption.Text"="Set [Nm]") -> ()  [unwired: 2 in, 2 out]
        n195 = Close File(refnum=w322, error in=w321) -> ()  [unwired: 2 out]
        n196 = local write "ARRAY IMPOSTAZIONI INV.FRENI"(w317) -> ()
        n197 = global read "BenchSelector.vi" "Bench Selector"() -> (w309:bool)
        n198 = Bundle By Name(cluster=T5 {"Message"="AGGIORNA SETTINGS FRENI", "Message Data"=variant} ("element"), "Message Data"=w317) -> (w331:T5)
        n199 = Select(t=0, s=w309, f=1) -> (s? t:f=w305:i32)
        n200 = Enqueue Element(queue=w327, element=w331) -> (queue out=w328:refnum<queue>, error out=w302:errorcluster)  [unwired: 2 in, 1 out]
        n201 = To Variant(anything=w305) -> (Variant=w306:variant)
        n202 = Bundle By Name(cluster=cluster{"Status":string, "variant":variant} {"Status"="Seleziona freno", "variant"=variant}, "variant"=w306) -> (w330:cluster{"Status":string, "variant":variant})
        n203 = Enqueue Element(queue=w328, element=w330, error in (no error)=w302) -> (queue out=w326:refnum<queue>, error out=w301:errorcluster)  [unwired: 1 in, 1 out]
        n204 = property on="Control Type" class="RadioBtnsControl (strict)"("Val(Sgnl)"=w315) -> ()  [unwired: 2 in, 2 out]
        n205 = global write "Global control type freno.vi" "Value"(w315) -> ()
        n206 = Enqueue Element(queue=w326, element=cluster{"Status":string, "variant":variant} {"Status"="REGOLA", "variant"=variant}, error in (no error)=w301) -> ()  [unwired: 1 in, 3 out]
      }
      frame "AGGIORNA SETTINGS FRENI" {
        n207 = Variant To Data(type=T4[] [{"Nome"="", "Cmax"=100.0, "Rpm max"=3000.0, "A max"=0.0, "Controllo RPM"={"PID gains Rpm"={"proportional gain (Kc)"=0.0, "integral time (Ti, min)"=0.0, "derivative time (Td, min)"=0.0}, "Abilita pid"=FALSE, "Precisione pid Rpm"=0.015, "Medie pid"=10, "Trampa[s]"=10, "Tstab ramp[s]"=10, "Max%pid"=10}, "Controllo coppia"={"PID gains Coppia"={"proportional gain (Kc)"=10.0, "integral time (Ti, min)"=0.015, "derivative time (Td, min)"=0.0}, "Abilita pid"=FALSE, "Precisione pid Nm"=0.0, "Medie pid"=0, "Trampa[s]"=0, "Tstab ramp[s]"=10, "Max%pid"=10}, "Controllo potenza"={"PID gains potenza"={"proportional gain (Kc)"=0.4, "integral time (Ti, min)"=0.025, "derivative time (Td, min)"=0.0}, "Abilita pid"=FALSE, "Precisione pid W"=0.015, "Medie pid"=10, "Trampa[s]"=10, "Tstab ramp[s]"=10, "Max%pid"=10}, "Compensa coppia residua"={"Abilita compensazione"=FALSE, "C residua [Nm]"=0.0, "C isteresi [Nm]"=0.0, "PID gains C-RPM"={"proportional gain (Kc)"=1.0, "integral time (Ti, min)"=0.01, "derivative time (Td, min)"=0.0}, "C precision [Nm]"=0.0, "Max%pid"=0, "Medie pid"=0}}, {"Nome"="", "Cmax"=200.0, "Rpm max"=4500.0, "A max"=0.0, "Controllo RPM"={"PID gains Rpm"={"proportional gain (Kc)"=0.0, "integral time (Ti, min)"=0.0, "derivative time (Td, min)"=0.0}, "Abilita pid"=FALSE, "Precisione pid Rpm"=0.015, "Medie pid"=10, "Trampa[s]"=10, "Tstab ramp[s]"=10, "Max%pid"=10}, "Controllo coppia"={"PID gains Coppia"={"proportional gain (Kc)"=10.0, "integral time (Ti, min)"=0.015, "derivative time (Td, min)"=0.0}, "Abilita pid"=FALSE, "Precisione pid Nm"=0.0, "Medie pid"=0, "Trampa[s]"=0, "Tstab ramp[s]"=10, "Max%pid"=10}, "Controllo potenza"={"PID gains potenza"={"proportional gain (Kc)"=0.4, "integral time (Ti, min)"=0.025, "derivative time (Td, min)"=0.0}, "Abilita pid"=FALSE, "Precisione pid W"=0.015, "Medie pid"=10, "Trampa[s]"=10, "Tstab ramp[s]"=10, "Max%pid"=10}, "Compensa coppia residua"={"Abilita compensazione"=FALSE, "C residua [Nm]"=0.0, "C isteresi [Nm]"=0.0, "PID gains C-RPM"={"proportional gain (Kc)"=1.0, "integral time (Ti, min)"=0.01, "derivative time (Td, min)"=0.0}, "C precision [Nm]"=0.0, "Max%pid"=0, "Medie pid"=0}}] ("ARRAY IMPOSTAZIONI INV.FRENI"), Variant=w354) -> (data=w345:T4[])  [unwired: 1 in, 1 out]
        n208 = global read "BenchSelector.vi" "Bench Selector"() -> (w343:bool)
        n209 = Array Size(array=w345) -> (size(s)=w348:i32)
        n210 = local write "ARRAY IMPOSTAZIONI INV.FRENI"(w345) -> ()
        n211 = Select(t=1 ("Freno selezionato"), s=w343, f=0) -> (s? t:f=w341:i32)
        n212 = To Variant(anything=w341) -> (Variant=w340:variant)
        n213 = Bundle By Name(cluster=cluster{"Status":string, "variant":variant} {"Status"="Seleziona freno", "variant"=variant}, "variant"=w340) -> (w352:cluster{"Status":string, "variant":variant})
        n214 = Enqueue Element(queue=w350, element=w352) -> ()  [unwired: 2 in, 3 out]
        n215 = Initialize Array(T1 {"DI senso rotaz freno"=FALSE, "Rif AO vel [RPM]"=0.0, "Rif AO coppia freno[Nm]"=0.0, "Abilitato"=FALSE, "Running"=FALSE, "Ctrl velocità"=FALSE, "Nome"="", "Ctrl coppia"=FALSE, "Impulso START"=FALSE, "Impulso STOP"=FALSE, "Rif AO Corr [A] "=0.0} ("Stato inverter"), w348) -> (w347:T1[])
        n216 = local write "Comandi freno"(w347) -> ()
      }
      frame "Aggiorna kw motore prova" {
        n217 = Variant To Data(type=0.0, Variant=w375) -> (data=w372:dbl)  [unwired: 1 in, 1 out]
        n218 = Equal To 0?(x=w372) -> (x = 0?=w370:bool)
        n219 = Not A Number/Path/Refnum?(number/path/refnum=w372) -> (NaN/Path/Refnum?=w371:bool)
        n220 = Or(x=w370, y=w371) -> (x .or. y?=w369:bool)
        n221 = Multiply(x=w372, y=1.5) -> (x*y=w368:dbl)
        n222 = Select(t=300.0, s=w369, f=w368) -> (s? t:f=w366:dbl)
        n223 = In Range and Coerce(upper limit=300.0, x=w366, lower limit=0.0) -> (coerced(x)=→"Kw Max prova":dbl)  [unwired: 1 out]
      }
      frame "Seleziona freno" {
        # "rpm nom?"
        n224 = Variant To Data(type=0, Variant=w413) -> (data=w405:i32)  [unwired: 1 in, 1 out]
        n225 = Index Array(array=w411, index=w405) -> (element=w402:T4)
        n226 = Unbundle By Name(w402) -> ("A max"=→"A max":dbl, "Cmax"=w392:dbl, "Rpm max"=w391:dbl, "Compensa coppia residua.Abilita compensazione"=w389:bool, "Controllo potenza.Precisione pid W"=w388:dbl, "Controllo coppia.Precisione pid Nm"=w387:dbl)  [unwired: 1 out]
        "Cmax" <- w392
        "Rpm max" <- w391
        n227 = property on="Compensazione velocità" class="Bool (strict)"("Visible"=w389, "Value"=FALSE ("Compensazione velocità")) -> ()  [unwired: 2 in, 2 out]
        n228 = property on="Comp." class="Bool (strict)"("Visible"=w389) -> ()  [unwired: 2 in, 2 out]
        n229 = local write "Precisione pid W"(w388) -> ()
        n230 = local write "Precisione pid Nm"(w387) -> ()
        n231 = Divide(x=w391, y=60.0) -> (x/y=w399:dbl)
        n232 = Multiply(x=w399, y=6.283185307179586) -> (x*y=w400:dbl)
        n233 = global write "Stato comandi freno.vi" "RPM max freno"(w391) -> ()
        n234 = Multiply(x=w400, y=w392) -> (x*y=w398:dbl)
        n235 = global write "Stato comandi freno.vi" "Cmax freno"(w392) -> ()
        n236 = Divide(x=w398, y=1000.0) -> (x/y=w397:dbl)
        n237 = Multiply(x=w397, y=0.95) -> (x*y=w401:dbl)
        n238 = local write "KW max banco"(w401) -> ()
      }
      frame "Aggiorna Cmax" {
        w417 = 3000.0  # rpm NOMINALI motore freno 2
        w418 = 3000.0  # rpm NOMINALI motore freno 1
        n239 = disable-structure shown="Enabled" {
          disable-tunnel: w428 -> [w439 _]
          disable-tunnel: [w438 w441] -> w421
          frame Disabled {
            n240 = Variant To Data(type=0.0, Variant=w439) -> (data=w438:dbl)  [unwired: 1 in, 1 out]
          }
          frame Enabled {
            n241 = local read "Cmax"() -> (w441:dbl)
          }
        }
        n242 = local write "Cmax"(w421) -> ()
        n243 = Build Array(w418, w417) -> (w416:dbl[])
        n244 = Index Array(array=w416, index=w415) -> (element=w414:dbl)
        n245 = Divide(x=w414, y=60.0) -> (x/y=w425:dbl)
        n246 = Multiply(x=w425, y=6.283185307179586) -> (x*y=w427:dbl)
        n247 = disable-structure shown="Enabled" {
          disable-tunnel: w419 -> [w444 w445]
          disable-tunnel: [w443 w445] -> w429
          disable-tunnel: w421 -> [w442 _]
          frame Disabled {
            n248 = Bundle By Name(cluster=w444, "Cmax"=w442) -> (w443:T4)
          }
          frame Enabled {
          }
        }
        n249 = Multiply(x=w427, y=w421) -> (x*y=w422:dbl)
        n250 = Divide(x=w422, y=1000.0) -> (x/y=→"KW max banco":dbl)
      }
      frame "Set C" {
        n251 = Variant To Data(type=0.0, Variant=w455) -> (data=w448:dbl)  [unwired: 1 in, 1 out]
        n252 = property on="Set" class="DigNum (strict)"("Value"=w448) -> ()  [unwired: 2 in, 2 out]
      }
      frame "Set Potenza" {
        n253 = Variant To Data(type=0.0, Variant=w469) -> (data=w461:dbl)  [unwired: 1 in, 1 out]
        n254 = property on="Set" class="DigNum (strict)"("Value"=w461) -> ()  [unwired: 2 in, 2 out]
        n255 = In Range and Coerce(upper limit=300.0, x=w461, lower limit=0.0) -> (coerced(x)=w460:dbl)  [unwired: 1 out]
      }
      frame "Set RPM" {
        n256 = Variant To Data(type=0.0, Variant=w481) -> (data=w473:dbl)  [unwired: 1 in, 1 out]
        n257 = property on="Set" class="DigNum (strict)"("Value"=w473) -> ()  [unwired: 2 in, 2 out]
      }
      frame "AGGIORNA COMANDI FRENO" {
        n258 = Variant To Data(type=T3 {"Control"={"Control Type"=enum."Torque [Nm]", "Set"=0.0, "Inverti senso di rotazione"=FALSE}, "Start\\stop"={"Start"=FALSE, "STOP"=FALSE}, "Status"={"Ready"=FALSE, "Running"=FALSE, "Regulation"=FALSE}, "PID"=FALSE, "Abilita"={"Abilita"=FALSE}, "Status ref"={"Torque"=0.0, "Speed"=0.0}} ("Gestione freno"), Variant=w505) -> (data=w494:T3)  [unwired: 1 in, 1 out]
        n259 = Unbundle By Name(w494) -> ("Control.Control Type"=w485:T2, "Control.Set"=w503:dbl, "PID"=w491:bool, "Start\\stop.Start"=w486:bool, "Start\\stop.STOP"=w489:bool, "Abilita.Abilita"=w495:bool, "Control.Inverti senso di rotazione"=w488:bool)
        "INVERTI SENSO ROT" <- w488
        n260 = local write "DO senso rotaz freno"(w488) -> ()
        n261 = local write "Gestione freno"(w494) -> ()
        n262 = Not(x=w489) -> (.not. x?=w487:bool)
        n263 = And(x=w487, y=w486) -> (x .and. y?=w490:bool)
        n264 = case shown="True" w490 {
          tunnel: w496 -> [_ w554]
          frame False {
          }
          frame True {
            n265 = Enqueue Element(queue=w554, element=cluster{"Status":string, "variant":variant} {"Status"="START", "variant"=variant}) -> ()  [unwired: 2 in, 3 out]
          }
        }
        n266 = case shown="True" w489 {
          tunnel: w496 -> [_ w552]
          frame False {
          }
          frame True {
            n267 = Enqueue Element(queue=w552, element=cluster{"Status":string, "variant":variant} {"Status"="STOP", "variant"=variant}) -> ()  [unwired: 2 in, 3 out]
          }
        }
        n268 = Not Equal?(x=w500, y=w485) -> (x != y?=w492:bool)
        n269 = global write "Global control type freno.vi" "Value"(w485) -> ()
        n270 = case shown="False" w492 {
          tunnel: w503 -> [w516 _]
          tunnel: w485 -> [w515 _]
          tunnel: w499 -> [w514 _]
          tunnel: w498 -> [w513 _]
          tunnel: w497 -> [w512 _]
          tunnel: w496 -> [w511 _]
          tunnel: [w510 _] -> w493
          frame False {
            n271 = case shown="\"Power [W]\"" w515 {
              tunnel: w516 -> [w520 w529 w539]
              tunnel: w511 -> [w521 w531 w541]
              tunnel: w514 -> [_ _ w540]
              tunnel: w513 -> [_ w530 _]
              tunnel: w512 -> [w519 _ _]
              tunnel: [w517 w527 w537] -> w510
              frame "Torque [Nm]", Default {
                n272 = Not Equal?(x=w520, y=w519) -> (x != y?=w518:bool)
                n273 = case shown="True" w518 {
                  tunnel: w520 -> [_ w524]
                  tunnel: w521 -> [_ w523]
                  tunnel: [_ w522] -> w517
                  frame False {
                  }
                  frame True {
                    n274 = Bundle By Name(cluster=cluster{"Status":string, "variant":variant} {"Status"="Set C", "variant"=variant}, "variant"=w524) -> (w526:cluster{"Status":string, "variant":variant})
                    n275 = Enqueue Element(queue=w523, element=w526) -> (error out=w522:errorcluster)  [unwired: 2 in, 2 out]
                  }
                }
              }
              frame "Power [W]" {
                n276 = Not Equal?(x=w529, y=w530) -> (x != y?=w528:bool)
                n277 = case shown="True" w528 {
                  tunnel: w531 -> [_ w534]
                  tunnel: w529 -> [_ w533]
                  tunnel: [_ w532] -> w527
                  frame False {
                  }
                  frame True {
                    n278 = Bundle By Name(cluster=cluster{"Status":string, "variant":variant} {"Status"="Set Potenza", "variant"=variant}, "variant"=w533) -> (w536:cluster{"Status":string, "variant":variant})
                    n279 = Enqueue Element(queue=w534, element=w536) -> (error out=w532:errorcluster)  [unwired: 2 in, 2 out]
                  }
                }
              }
              frame "Speed [RPM]" {
                n280 = Not Equal?(x=w539, y=w540) -> (x != y?=w538:bool)
                n281 = case shown="True" w538 {
                  tunnel: w541 -> [_ w544]
                  tunnel: w539 -> [_ w543]
                  tunnel: [_ w542] -> w537
                  frame False {
                  }
                  frame True {
                    n282 = Bundle By Name(cluster=cluster{"Status":string, "variant":variant} {"Status"="Set RPM", "variant"=variant}, "variant"=w543) -> (w546:cluster{"Status":string, "variant":variant})
                    n283 = Enqueue Element(queue=w544, element=w546) -> (error out=w542:errorcluster)  [unwired: 2 in, 2 out]
                  }
                }
              }
            }
          }
          frame True {
          }
        }
        n284 = case shown="True" w492 {
          tunnel: w496 -> [_ w557]
          tunnel: w485 -> [_ w556]
          tunnel: w493 -> [_ w555]
          frame False {
          }
          frame True {
            n285 = Bundle By Name(cluster=cluster{"Status":string, "variant":variant} {"Status"="Set tipo controllo", "variant"=variant}, "variant"=w556) -> (w558:cluster{"Status":string, "variant":variant})
            n286 = Enqueue Element At Opposite End(queue=w557, element=w558, error in (no error)=w555) -> ()  [unwired: 1 in, 3 out]
          }
        }
        n287 = case shown="False" w495 {
          tunnel: w496 -> [w547 w550]
          frame False {
            n288 = Enqueue Element(queue=w547, element=cluster{"Status":string, "variant":variant} {"Status"="DISABILITA", "variant"=variant}) -> ()  [unwired: 2 in, 3 out]
          }
          frame True {
            n289 = Enqueue Element(queue=w550, element=cluster{"Status":string, "variant":variant} {"Status"="ABILITA", "variant"=variant}) -> ()  [unwired: 2 in, 3 out]
          }
        }
        n290 = Bundle By Name(cluster=w502, "Controllo coppia.Abilita pid"=w491, "Controllo potenza.Abilita pid"=w491, "Controllo RPM.Abilita pid"=w491) -> (w501:T4)
      }
      frame "ABILITA" {
        "Abilita" <- TRUE
      }
      frame "DISABILITA" {
        n291 = local write "Abilita"(FALSE ("Boolean")) -> ()
      }
      frame "IDLE" {
      }
      frame "START" {
        w593 = T2."Torque [Nm]" ("Value")
        # "è possibile partire solo in \ntipo controllo coppia"
        n292 = local read "Array stato inverter freno"() -> (w599:T1[])
        n293 = Index Array(array=w599, index=w597) -> (element=w598:T1)
        n294 = Unbundle By Name(w598) -> ("Running"=w595:bool)
        n295 = control-ref of="Control Type"() -> (w592:refnum<vi>)
        n296 = Equal?(x=w601, y=w593) -> (x = y?=w596:bool)
        n297 = Or(x=w596, y=w595) -> (x .or. y?=w594:bool)
        n298 = case shown="True" w594 {
          tunnel: w593 -> [w613 _]
          tunnel: w600 -> [w612 _]
          tunnel: w592 -> [_ w617]
          frame False {
            n299 = Bundle By Name(cluster=cluster{"Status":string, "variant":variant} {"Status"="Set tipo controllo", "variant"=variant}, "variant"=w613) -> (w615:cluster{"Status":string, "variant":variant})
            n300 = Enqueue Element At Opposite End(queue=w612, element=w615) -> (queue out=w611:refnum<queue>)  [unwired: 2 in, 2 out]
            n301 = Enqueue Element(queue=w611, element=T5 {"Message"="START", "Message Data"=variant}) -> ()  [unwired: 2 in, 3 out]
          }
          frame True {
            n302 = property on="Start" class="Bool (strict)"("Value"=FALSE) -> ()  [unwired: 2 in, 2 out]
            n303 = property class="RadioBtnsControl (strict)"(reference=w617, "DisabledEnum"=T42."Disabled and Grayed Out" ("Disabled")) -> ()  [unwired: 1 in, 2 out]
            "start" <- TRUE ("Boolean")
          }
        }
      }
      frame "STOP" {
        n304 = control-ref of="Control Type"() -> (w621:refnum<vi>)
        n305 = property class="RadioBtnsControl (strict)"(reference=w621, "DisabledEnum"=T42."Enabled" ("Disabled")) -> ()  [unwired: 1 in, 2 out]
        n306 = flat-sequence {
          frame #0 {
            n307 = local write "start"(FALSE ("Boolean")) -> ()
            n308 = property on="STOP" class="Bool (strict)"("Value"=FALSE) -> ()  [unwired: 2 in, 2 out]
          }
          frame #1 {
            n309 = Wait (ms)(milliseconds to wait=u32 2000) -> ()  [unwired: 1 out]
          }
          frame #2 {
            n310 = property on="Control Type" class="RadioBtnsControl (strict)"("Val(Sgnl)"=T2."Torque [Nm]" ("Value")) -> ()  [unwired: 2 in, 2 out]
          }
        }
        n311 = local write "Rif % AO RPM"(0.0 ("Rif % AO RPM")) -> ()
      }
      frame "Set tipo controllo" {
        n312 = Variant To Data(type=T2."Torque [Nm]" ("Value"), Variant=w668) -> (data=w638:T2)  [unwired: 1 in, 1 out]
        n313 = Unbundle By Name(w656) -> ("COPPIA"=w653:dbl, "POTENZA"=w651:dbl, "RPM"=w650:dbl)
        n314 = Equal?(x=w664, y=T2."Torque [Nm]" ("Value")) -> (x = y?=w666:bool)
        n315 = Equal?(x=w664, y=T2."Power [W]" ("Value")) -> (x = y?=w667:bool)
        n316 = Equal?(x=w638, y=T2."Speed [RPM]" ("Value")) -> (x = y?=w662:bool)
        n317 = Equal?(x=w638, y=T2."Torque [Nm]" ("Value")) -> (x = y?=w661:bool)
        n318 = Equal?(x=w638, y=T2."Power [W]" ("Value")) -> (x = y?=w660:bool)
        n319 = Divide(x=w651, y=1000.0) -> (x/y=w646:dbl)
        n320 = Or(x=w666, y=w667) -> (x .or. y?=w658:bool)
        n321 = Or(x=w661, y=w660) -> (x .or. y?=w659:bool)
        n322 = And(x=w658, y=w659) -> (x .and. y?=w657:bool)
        n323 = Index Array(array=string[] ["Set [Nm]", "Set [kW]", "Set [RPM]", "Set [A]"], index=w638) -> (element=w647:string)
        n324 = case shown="\"Speed [RPM]\"" w638 {
          tunnel: w653 -> [w675 _ _]
          tunnel: [w675 w676 w677] -> w652
          tunnel: w646 -> [_ w676 _]
          tunnel: w650 -> [_ _ w677]
          frame "Torque [Nm]", Default {
          }
          frame "Power [W]" {
          }
          frame "Speed [RPM]" {
          }
        }
        n325 = property on="Control Type" class="RadioBtnsControl (strict)"("Value"=w638) -> ()  [unwired: 2 in, 2 out]
        n326 = property on="Set" class="DigNum (strict)"("Caption.Text"=w647) -> ()  [unwired: 2 in, 2 out]
        n327 = Select(t=w638, s=w657, f=w664) -> (s? t:f=w663:T2)
        n328 = case shown="True" w657 {
          tunnel: w649 -> [w679 w687]
          tunnel: w662 -> [w678 _]
          frame False {
            n329 = case shown="False" w678 {
              tunnel: w679 -> [w681 w684]
              frame False {
                n330 = Flush Queue(queue=w681) -> (queue out=w680:refnum<queue>)  [unwired: 1 in, 2 out]
                n331 = Enqueue Element At Opposite End(queue=w680, element=T5 {"Message"="Passaggio velocità coppia", "Message Data"=variant}) -> ()  [unwired: 2 in, 3 out]
              }
              frame True {
                n332 = Flush Queue(queue=w684) -> (queue out=w683:refnum<queue>)  [unwired: 1 in, 2 out]
                n333 = Enqueue Element At Opposite End(queue=w683, element=T5 {"Message"="Passaggio coppia velocità", "Message Data"=variant}) -> ()  [unwired: 2 in, 3 out]
              }
            }
          }
          frame True {
            n334 = global write "Global CAMBIO CTRL FRENO.vi" "CAMBIO CTRL IN CORSO"(FALSE ("CAMBIO CTRL IN CORSO")) -> ()
            n335 = Enqueue Element At Opposite End(queue=w687, element=T5 {"Message"="REGOLA", "Message Data"=variant}) -> ()  [unwired: 2 in, 3 out]
          }
        }
        n336 = case shown="\"Power [W]\"" w638 {
          tunnel: [T7[] [{"DO"=enum."Select current mode", "Value"=FALSE}, {"DO"=enum."Select speed mode", "Value"=FALSE}, {"DO"=enum."Select torque mode", "Value"=TRUE}] T7[] [{"DO"=enum."Select current mode", "Value"=FALSE}, {"DO"=enum."Select torque mode", "Value"=TRUE}, {"DO"=enum."Select speed mode", "Value"=FALSE}] T7[] [{"DO"=enum."Select current mode", "Value"=FALSE}, {"DO"=enum."Select torque mode", "Value"=FALSE}, {"DO"=enum."Select speed mode", "Value"=TRUE}] T7[] [{"DO"=enum."Select speed mode", "Value"=FALSE}, {"DO"=enum."Select torque mode", "Value"=FALSE}, {"DO"=enum."Select current mode", "Value"=TRUE}]] -> w637
          frame "Torque [Nm]", Default {
          }
          frame "Power [W]" {
          }
          frame "Speed [RPM]" {
          }
          frame "Corrente [A]" {
          }
        }
        n337 = property on="Set" class="DigNum (strict)"("Value"=w652) -> ()  [unwired: 2 in, 2 out]
        n338 = call "Set DO.vi"("Cluster SET DO"=w637) -> ()  [unwired: 10 in, 1 out]
      }
      frame "Ctrl velocità disponibile" {
        n339 = Variant To Data(type=TRUE, Variant=w691) -> ()  [unwired: 1 in, 2 out]
        n340 = property on="Speed [RPM]" class="Bool (strict)"("Visible"=TRUE) -> ()  [unwired: 2 in, 2 out]
      }
      frame "Passaggio coppia velocità" {
        # "ATTENZIONE AL SENSO DI ROTAZIONE nel case \"Verifica senso di rotazione\"."
        n341 = Wait Until Next ms Multiple(millisecond multiple=w707) -> ()  [unwired: 1 out]
        n342 = case shown="False" TRUE {
          tunnel: w719 -> [w728 w830]
          tunnel: w718 -> [w727 w829]
          tunnel: w717 -> [w726 w828]
          tunnel: [w725 w827] -> w716
          tunnel: [w724 w826] -> w713
          tunnel: [w723 w825] -> w710
          tunnel: w709 -> [w722 w824]
          tunnel: w705 -> [w721 w823]
          tunnel: [w720 _] -> w702
          frame True {
            n343 = while {
              shift-right: [w739] -> w723
              shift-left: w721 -> [w740]
              tunnel: w728 -> [w738]
              tunnel: w727 -> [w737]
              shift-right: [w735] -> w725
              shift-left: w726 -> [w736]
              tunnel: [w734] -> w724
              tunnel: w722 -> [w733]
              shift-right: [w732] -> w720
              shift-left: _ -> [w731]
              shift-right: [w730] -> _
              shift-left: _ -> [w729]
              stop <- TRUE stop-if-true
              n344 = case shown="\"Set riferimento di velocità iniziale\"" w740 {
                selector: w740 -> [w761 w782 w810 w822]
                tunnel: [w760 w781 w809 w822] -> w739
                tunnel: w738 -> [w756 _ _ _]
                tunnel: w737 -> [_ w795 _ _]
                tunnel: [w744 w780 w807 T2."Speed [RPM]" ("Value")] -> w735
                tunnel: w736 -> [w744 w780 w807 _]
                tunnel: [_ _ _ TRUE] -> w734
                tunnel: w733 -> [w750 w769 w798 _]
                tunnel: [w755 w773 w799 w819] -> w732
                tunnel: w731 -> [_ w773 w799 w819]
                tunnel: [TRUE _ _ _] -> w730
                tunnel: w729 -> [_ w770 _ _]
                frame "Verifica senso di rotazione", Default {
                  # "ATTENZIONE AL BIT SENSO DI ROTAZIONE. Impostarlo in modo da avere una\nrotazione concorde con il verso attuale."
                  n345 = global read "Global_All_Data.vi" "All Data"() -> (w753:T11)
                  n346 = Unbundle By Name(w753) -> ("MISURE ALL.STATO PLC 1.AI plc.RPM freno"=w749:dbl, "MISURE ALL.STATO PLC 3.AI plc.RPM freno"=w748:dbl)
                  n347 = Unbundle By Name(w756) -> ("RPM"=w757:dbl)
                  n348 = flat-sequence {
                    tunnel: w745 -> [w762]
                    tunnel: [w764] -> w758
                    tunnel: w750 -> [w766]
                    frame #0 {
                      n349 = property on="Inverti senso di rotazione" class="Bool (strict)"("Value"=w762) -> ()  [unwired: 2 in, 2 out]
                      "DO senso rotaz freno" <- w762
                    }
                    frame #1 {
                      n350 = local read "Comandi freno"() -> (w767:T1[])
                      n351 = Index Array(array=w767, index=w766) -> (element=w765:T1)
                      n352 = local write "INVERTI SENSO ROT"(FALSE ("iNVERTI SENSO ROT")) -> ()
                      n353 = Unbundle By Name(w765) -> ("DI senso rotaz freno"=w764:bool)
                    }
                  }
                  n354 = Absolute Value(x=w757) -> (abs(x)=w755:dbl)
                  n355 = Greater Or Equal To 0?(x=w749) -> (x >= 0?=w752:bool)
                  n356 = Greater Or Equal To 0?(x=w748) -> (x >= 0?=w743:bool)
                  n357 = Not(x=w752) -> (.not. x?=w747:bool)
                  n358 = Not(x=w743) -> (.not. x?=w742:bool)
                  n359 = Build Array(w747, w742) -> (w746:bool[])
                  n360 = Index Array(array=w746, index=w750) -> (element=w745:bool)
                  n361 = Equal?(x=w758, y=w745) -> (x = y?=w754:bool)
                  n362 = Select(t="Set riferimento di velocità iniziale", s=w754, f=w761) -> (s? t:f=w760:string)
                }
                frame "Set riferimento di velocità iniziale" {
                  n363 = Unbundle By Name(w795) -> ("Rpm max"=w776:dbl)
                  n364 = local read "Array stato inverter freno"() -> (w778:T1[])
                  n365 = Index Array(array=w778, index=w769) -> (element=w779:T1)
                  n366 = Unbundle By Name(w779) -> ("Rif AO vel [RPM]"=w777:dbl)
                  n367 = Divide(x=w773, y=w776) -> (x/y=w791:dbl)
                  n368 = Multiply(x=w791, y=100.0) -> (x*y=w775:dbl)
                  n369 = Multiply(x=w773, y=1.05) -> (x*y=w787:dbl)
                  n370 = Multiply(x=w773, y=0.95) -> (x*y=w785:dbl)
                  n371 = Absolute Value(x=w777) -> (abs(x)=w774:dbl)
                  n372 = In Range and Coerce(upper limit=100.0, x=w775, lower limit=0.0) -> ()  [unwired: 2 out]
                  n373 = In Range and Coerce(upper limit=w787, x=w774, lower limit=w785) -> (In Range?=w789:bool)  [unwired: 1 out]
                  n374 = Not(x=w789) -> (.not. x?=w790:bool)
                  n375 = Or(x=w790, y=w770) -> (x .or. y?=w771:bool)
                  n376 = call "Elapsed Time"("Time Target (s)"=2.5, "Reset"=w771, "Auto Reset"=FALSE) -> ("Time has Elapsed"=w783:bool)  [unwired: 9 in, 7 out]
                  n377 = Select(t="Rif coppia max", s=w783, f=w782) -> (s? t:f=w781:string)
                  "Rif AO vel [RPM]" <- w773
                }
                frame "Rif coppia max" {
                  n378 = Equal?(x=w798, y=1) -> (x = y?=w796:bool)
                  n379 = disable-structure shown="Enabled" {
                    disable-tunnel: [w815 4000.0 ("%Rif AO coppia freno")] -> w802
                    disable-tunnel: w796 -> [w814 _]
                    frame Enabled {
                      # "400% SANTERNO\n100% KEB"
                      n380 = local read "Cmax"() -> (w816:dbl)
                      n381 = Select(t=1.0 ("y"), s=w814, f=4.0 ("y")) -> (s? t:f=w811:dbl)
                      n382 = Multiply(x=w816, y=w811) -> (x*y=w815:dbl)
                    }
                    frame Disabled {
                    }
                  }
                  "Rif AO coppia freno [Nm]" <- w802
                  n383 = local read "Comandi freno"() -> (w805:T1[])
                  n384 = Index Array(array=w805, index=w798) -> (element=w806:T1)
                  n385 = Unbundle By Name(w806) -> ("Rif AO coppia freno[Nm]"=w804:dbl)
                  n386 = Increment(x=w802) -> (x+1=w803:dbl)
                  n387 = Decrement(x=w802) -> (x-1=w801:dbl)
                  n388 = In Range and Coerce(upper limit=w803, x=w804, lower limit=w801) -> (In Range?=w800:bool)  [unwired: 1 out]
                  n389 = Select(t="Fine impostazioni controllo velocità", s=w800, f=w810) -> (s? t:f=w809:string)
                }
                frame "Fine impostazioni controllo velocità" {
                  n390 = global write "Global CAMBIO CTRL FRENO.vi" "CAMBIO CTRL IN CORSO"(FALSE ("CAMBIO CTRL IN CORSO")) -> ()
                }
              }
            }
          }
          frame False {
            n391 = disable-structure shown="Disabled" {
              disable-tunnel: w830 -> [w838 _]
              disable-tunnel: w829 -> [w837 _]
              disable-tunnel: w828 -> [w836 _]
              disable-tunnel: [w835 _] -> w827
              disable-tunnel: [w834 _] -> w826
              disable-tunnel: [w833 _] -> w825
              disable-tunnel: w824 -> [w832 _]
              disable-tunnel: w823 -> [w831 _]
              frame Disabled {
                # "per pentair"
                n392 = while {
                  shift-right: [w847] -> w833
                  shift-left: w831 -> [w848]
                  tunnel: w838 -> [w846]
                  tunnel: w837 -> [w845]
                  shift-right: [w843] -> w835
                  shift-left: w836 -> [w844]
                  tunnel: [w842] -> w834
                  tunnel: w832 -> [w841]
                  shift-right: [w840] -> _
                  shift-left: _ -> [w839]
                  stop <- TRUE stop-if-true
                  n393 = case shown="\"Set riferimento di velocità iniziale\"" w848 {
                    selector: w848 -> [w860 w864 w874 w894 w907 w927 w934 w942 w950]
                    tunnel: [w859 w865 w873 w893 w906 w926 w933 w941 w950] -> w847
                    tunnel: w846 -> [w862 _ _ _ _ _ _ _ _]
                    tunnel: w845 -> [_ _ _ _ w921 _ _ _ _]
                    tunnel: [w857 w870 w882 w892 w905 w923 w931 w939 T44."Speed [RPM]" ("Control Type")] -> w843
                    tunnel: w844 -> [w857 w870 w882 w892 w905 w923 w931 w939 _]
                    tunnel: [_ _ _ _ _ _ _ _ TRUE] -> w842
                    tunnel: w841 -> [w853 _ w881 w889 w902 _ _ _ _]
                    tunnel: [w852 w863 w872 w886 w897 w922 w930 w938 w947] -> w840
                    tunnel: w839 -> [_ w863 w872 w886 w897 w922 w930 w938 w947]
                    frame "Verifica senso di rotazione", Default {
                      n394 = local read "Array stato inverter freno"() -> (w855:T1[])
                      n395 = global read "Global senso rotazione.vi" "Senso rot (T<0 F>0)"() -> (w851:bool)
                      n396 = Unbundle By Name(w862) -> ("RPM"=w852:dbl)
                      n397 = Index Array(array=w855, index=w853) -> (element=w856:T1)
                      n398 = Less Than 0?(x=w852) -> ()  [unwired: 1 out]
                      n399 = Unbundle By Name(w856) -> ("DI senso rotaz freno"=w854:bool)
                      n400 = Not(x=w851) -> (.not. x?=w850:bool)
                      n401 = Equal?(x=w854, y=w850) -> (x = y?=w861:bool)
                      n402 = local write "DO senso rotaz freno"(w850) -> ()
                      n403 = Select(t="Azionamento in blocco", s=w861, f=w860) -> (s? t:f=w859:string)
                    }
                    frame "Azionamento in blocco" {
                      n404 = global read "Global_All_Data.vi" "All Data"() -> (w868:T11)
                      n405 = Unbundle By Name(w868) -> ("Abilita AFE"=w867:bool)
                      n406 = call "Set DO.vi"("Cluster SET DO"=T43 [{"DO"=enum."Comando azionam in blocco", "Value"=TRUE}]) -> ()  [unwired: 10 in, 1 out]
                      n407 = Select(t="Togli controlli", s=w867, f=w864) -> (s? t:f=w865:string)
                    }
                    frame "Togli controlli" {
                      w876 = FALSE ("Ctrl velocità")
                      n408 = local read "Array stato inverter freno"() -> (w883:T1[])
                      n409 = Index Array(array=w883, index=w881) -> (element=w884:T1)
                      n410 = Unbundle By Name(w884) -> ("Ctrl velocità"=w880:bool, "Ctrl coppia"=w879:bool)
                      n411 = Not(x=w880) -> (.not. x?=w877:bool)
                      n412 = Not(x=w879) -> (.not. x?=w878:bool)
                      n413 = And(x=w877, y=w878) -> (x .and. y?=w875:bool)
                      n414 = Select(t="Set controllo velocità", s=w875, f=w874) -> (s? t:f=w873:string)
                      "Ctrl velocità" <- w876
                      "Ctrl coppia" <- w876
                    }
                    frame "Set controllo velocità" {
                      n415 = local read "Array stato inverter freno"() -> (w890:T1[])
                      n416 = Index Array(array=w890, index=w889) -> (element=w891:T1)
                      n417 = local write "Ctrl velocità"(TRUE ("Ctrl velocità")) -> ()
                      n418 = Unbundle By Name(w891) -> ("Ctrl velocità"=w887:bool)
                      n419 = Select(t="Set riferimento di velocità iniziale", s=w887, f=w894) -> (s? t:f=w893:string)
                    }
                    frame "Set riferimento di velocità iniziale" {
                      n420 = Unbundle By Name(w921) -> ("Rpm max"=w900:dbl)
                      n421 = local read "Array stato inverter freno"() -> (w903:T1[])
                      n422 = Index Array(array=w903, index=w902) -> (element=w904:T1)
                      n423 = Unbundle By Name(w904) -> ("Rif AO vel [RPM]"=w901:dbl)
                      n424 = Absolute Value(x=w897) -> (abs(x)=w898:dbl)
                      n425 = Divide(x=w898, y=w900) -> (x/y=w917:dbl)
                      n426 = Multiply(x=w917, y=100.0) -> (x*y=w899:dbl)
                      n427 = Absolute Value(x=w901) -> (abs(x)=w895:dbl)
                      n428 = Multiply(x=w898, y=1.05) -> (x*y=w911:dbl)
                      n429 = Multiply(x=w898, y=0.95) -> (x*y=w909:dbl)
                      n430 = In Range and Coerce(upper limit=100.0, x=w899, lower limit=0.0) -> ()  [unwired: 2 out]
                      n431 = In Range and Coerce(upper limit=w911, x=w895, lower limit=w909) -> (In Range?=w913:bool)  [unwired: 1 out]
                      n432 = local write "Rif AO vel [RPM]"(w898) -> ()
                      n433 = Not(x=w913) -> (.not. x?=w914:bool)
                      n434 = call "Elapsed Time2"("Time Target (s)"=2.0, "Reset"=w914, "Auto Reset"=FALSE) -> ("Time has Elapsed"=w908:bool)  [unwired: 9 in, 7 out]
                      n435 = Select(t="Togli blocco azionamento", s=w908, f=w907) -> (s? t:f=w906:string)
                    }
                    frame "Togli blocco azionamento" {
                      n436 = global read "Global_All_Data.vi" "All Data"() -> (w928:T11)
                      n437 = Unbundle By Name(w928) -> ("Abilita AFE"=w924:bool)
                      n438 = call "Set DO.vi"("Cluster SET DO"=T43 [{"DO"=enum."Comando azionam in blocco", "Value"=FALSE}]) -> ()  [unwired: 10 in, 1 out]
                      n439 = Select(t=w927, s=w924, f="Comando azionamento reset" ("t")) -> (s? t:f=w926:string)
                    }
                    frame "Comando azionamento reset" {
                      n440 = global read "Global_All_Data.vi" "All Data"() -> (w936:T11)
                      n441 = Unbundle By Name(w936) -> ("MISURE ALL.STATO PLC 1.USCITE PLC.DO (bit).Reset allarmi"=w935:bool)
                      n442 = call "Set DO.vi"("Cluster SET DO"=T43 [{"DO"=enum."Comando azionam reset", "Value"=TRUE}]) -> ()  [unwired: 10 in, 1 out]
                      n443 = Select(t="Togli reset", s=w935, f=w934) -> (s? t:f=w933:string)
                    }
                    frame "Togli reset" {
                      n444 = global read "Global_All_Data.vi" "All Data"() -> (w944:T11)
                      n445 = Unbundle By Name(w944) -> ("MISURE ALL.STATO PLC 1.USCITE PLC.DO (bit).Reset allarmi"=w943:bool)
                      n446 = call "Set DO.vi"("Cluster SET DO"=T43 [{"DO"=enum."Comando azionam reset", "Value"=FALSE}]) -> ()  [unwired: 10 in, 1 out]
                      n447 = Select(t=w942, s=w943, f="Fine impostazioni controllo velocità" ("t")) -> (s? t:f=w941:string)
                    }
                    frame "Fine impostazioni controllo velocità" {
                      n448 = global write "Global CAMBIO CTRL FRENO.vi" "CAMBIO CTRL IN CORSO"(FALSE ("CAMBIO CTRL IN CORSO")) -> ()
                    }
                  }
                }
              }
              frame Enabled {
              }
            }
          }
        }
        n449 = case shown="False" w713 {
          tunnel: w714 -> [w951 w955]
          frame False {
            n450 = Enqueue Element(queue=w951, element=cluster{"Status":string, "variant":variant} {"Status"="Passaggio coppia velocità", "variant"=variant}) -> ()  [unwired: 2 in, 3 out]
          }
          frame True {
            n451 = Flush Queue(queue=w955) -> (queue out=w953:refnum<queue>)  [unwired: 1 in, 2 out]
            n452 = Enqueue Element At Opposite End(queue=w953, element=cluster{"Status":string, "variant":variant} {"Status"="REGOLA", "variant"=variant}) -> ()  [unwired: 2 in, 3 out]
          }
        }
      }
      frame "Passaggio velocità coppia" {
        n453 = Unbundle By Name(w972) -> ("RPM"=w971:dbl)
        n454 = Unbundle By Name(w958) -> ("Cmax"=w969:dbl)
        n455 = Wait Until Next ms Multiple(millisecond multiple=w960) -> ()  [unwired: 1 out]
        n456 = case shown="True" TRUE {
          tunnel: w973 -> [w986 w1061]
          tunnel: w971 -> [w985 w1060]
          tunnel: w970 -> [w984 w1059]
          tunnel: w969 -> [w983 w1058]
          tunnel: w968 -> [w982 w1057]
          tunnel: w967 -> [w981 w1056]
          tunnel: [w980 w1055] -> w966
          tunnel: [w979 w1054] -> w964
          tunnel: [w978 w1053] -> w963
          tunnel: w962 -> [w977 w1052]
          tunnel: w961 -> [w976 w1051]
          frame True {
            n457 = while {
              shift-right: [w992] -> w978
              shift-left: w977 -> [w997]
              tunnel: w986 -> [w996]
              tunnel: w985 -> [w995]
              tunnel: w984 -> [w994]
              tunnel: w983 -> [w993]
              shift-right: [w989] -> w980
              shift-left: w981 -> [w991]
              tunnel: w982 -> [w990]
              tunnel: [w988] -> w979
              tunnel: w976 -> [w987]
              stop <- TRUE stop-if-true
              n458 = case shown="\"Set rif vel a 0\"" w997 {
                selector: w997 -> [w1009 w1041 w1050]
                tunnel: w996 -> [w1023 _ _]
                tunnel: w995 -> [w1022 _ _]
                tunnel: w994 -> [w1021 _ _]
                tunnel: w993 -> [w1015 _ _]
                tunnel: [w1008 w1040 w1050] -> w992
                tunnel: w991 -> [w1005 w1038 _]
                tunnel: w990 -> [w1006 _ w1049]
                tunnel: [w1005 w1038 w1049] -> w989
                tunnel: [_ _ TRUE] -> w988
                tunnel: w987 -> [w1001 w1034 _]
                frame "Set rif coppia", Default {
                  n459 = case shown="\"Torque [Nm]\", Default" w1006 {
                    tunnel: w1023 -> [w1026 _ _]
                    tunnel: [w1025 w1031 _] -> w1000
                    tunnel: w1022 -> [_ w1032 _]
                    tunnel: w1021 -> [_ w1030 _]
                    frame "Torque [Nm]", Default {
                      n460 = Less Than 0?(x=w1026) -> (x < 0?=w1027:bool)
                      n461 = Select(t=0.0, s=w1027, f=w1026) -> (s? t:f=w1025:dbl)
                    }
                    frame "Power [W]" {
                      n462 = Multiply(x=w1030, y=1000.0) -> (x*y=w1028:dbl)
                      n463 = call "Coppia da potenza.vi"("Pmecc W"=w1028, "RPM letti"=w1032) -> ("t"=w1031:dbl)  [unwired: 9 in]
                    }
                    frame "Speed [RPM]" {
                    }
                  }
                  n464 = local read "Comandi freno"() -> (w1003:T1[])
                  n465 = Index Array(array=w1003, index=w1001) -> (element=w1004:T1)
                  n466 = Unbundle By Name(w1004) -> ("Rif AO coppia freno[Nm]"=w1002:dbl)
                  n467 = Divide(x=w1000, y=w1015) -> (x/y=w1017:dbl)
                  n468 = Absolute Value(x=w1000) -> (abs(x)=w999:dbl)
                  n469 = Multiply(x=w1017, y=100.0) -> (x*y=w1019:dbl)
                  n470 = In Range and Coerce(upper limit=100.0, x=w1019, lower limit=0.0) -> ()  [unwired: 2 out]
                  n471 = local write "Rif AO coppia freno [Nm]"(w999) -> ()
                  n472 = Multiply(x=0.9, y=w999) -> (x*y=w1011:dbl)
                  n473 = Multiply(x=1.1, y=w999) -> (x*y=w1013:dbl)
                  n474 = In Range and Coerce(upper limit=w1013, x=w1002, lower limit=w1011) -> (In Range?=w1010:bool)  [unwired: 1 out]
                  n475 = Select(t="Set rif vel a 0", s=w1010, f=w1009) -> (s? t:f=w1008:string)
                }
                frame "Set rif vel a 0" {
                  w1033 = 0.0 ("y")
                  n476 = local read "Array stato inverter freno"() -> (w1036:T1[])
                  n477 = Index Array(array=w1036, index=w1034) -> (element=w1037:T1)
                  n478 = Unbundle By Name(w1037) -> ("Rif AO vel [RPM]"=w1035:dbl)
                  n479 = Multiply(x=0.99, y=w1033) -> (x*y=w1043:dbl)
                  n480 = Multiply(x=1.01, y=w1033) -> (x*y=w1045:dbl)
                  n481 = In Range and Coerce(upper limit=w1045, x=w1035, lower limit=w1043) -> (In Range?=w1042:bool)  [unwired: 1 out]
                  n482 = local write "Rif AO vel [RPM]"(w1033) -> ()
                  n483 = Select(t="Fine imposta controllo coppia", s=w1042, f=w1041) -> (s? t:f=w1040:string)
                }
                frame "Fine imposta controllo coppia" {
                  n484 = global write "Global CAMBIO CTRL FRENO.vi" "CAMBIO CTRL IN CORSO"(FALSE ("CAMBIO CTRL IN CORSO")) -> ()
                }
              }
            }
          }
          frame False {
            n485 = disable-structure shown="Disabled" {
              disable-tunnel: w1061 -> [w1072 _]
              disable-tunnel: w1060 -> [w1071 _]
              disable-tunnel: w1059 -> [w1070 _]
              disable-tunnel: w1058 -> [w1069 _]
              disable-tunnel: w1057 -> [w1068 _]
              disable-tunnel: w1056 -> [w1067 _]
              disable-tunnel: [w1066 _] -> w1055
              disable-tunnel: [w1065 _] -> w1054
              disable-tunnel: [w1064 _] -> w1053
              disable-tunnel: w1052 -> [w1063 _]
              disable-tunnel: w1051 -> [w1062 _]
              frame Disabled {
                # "per pentair"
                n486 = while {
                  shift-right: [w1078] -> w1064
                  shift-left: w1063 -> [w1083]
                  tunnel: w1072 -> [w1082]
                  tunnel: w1071 -> [w1081]
                  tunnel: w1070 -> [w1080]
                  tunnel: w1069 -> [w1079]
                  shift-right: [w1075] -> w1066
                  shift-left: w1067 -> [w1077]
                  tunnel: w1068 -> [w1076]
                  tunnel: [w1074] -> w1065
                  tunnel: w1062 -> [w1073]
                  stop <- TRUE stop-if-true
                  n487 = case shown="\"Set rif coppia\"" w1083 {
                    selector: w1083 -> [w1088 w1099 w1113 w1125 w1147 w1153 w1159 w1168]
                    tunnel: w1082 -> [_ _ _ w1139 _ _ _ _]
                    tunnel: w1081 -> [_ _ _ w1138 _ _ _ _]
                    tunnel: w1080 -> [_ _ _ w1137 _ _ _ _]
                    tunnel: w1079 -> [_ _ _ w1131 _ _ _ _]
                    tunnel: [w1087 w1093 w1112 w1124 w1146 w1152 w1160 w1168] -> w1078
                    tunnel: w1077 -> [w1085 w1092 w1111 w1121 w1150 w1157 w1164 _]
                    tunnel: w1076 -> [_ _ _ w1122 _ _ _ w1167]
                    tunnel: [w1085 w1092 w1111 w1121 w1150 w1157 w1164 w1167] -> w1075
                    tunnel: [_ _ _ _ _ _ _ TRUE] -> w1074
                    tunnel: w1073 -> [_ w1101 w1108 w1117 _ _ _ _]
                    frame "Azionamento in blocco", Default {
                      n488 = global read "Global_All_Data.vi" "All Data"() -> (w1090:T11)
                      n489 = Unbundle By Name(w1090) -> ("Abilita AFE"=w1089:bool)
                      n490 = call "Set DO.vi"("Cluster SET DO"=T43 [{"DO"=enum."Comando azionam in blocco", "Value"=TRUE}]) -> ()  [unwired: 10 in, 1 out]
                      n491 = Select(t="Togli controlli", s=w1089, f=w1088) -> (s? t:f=w1087:string)
                    }
                    frame "Togli controlli" {
                      w1104 = FALSE ("Ctrl velocità")
                      n492 = local write "Ctrl velocità"(w1104) -> ()
                      n493 = local write "Ctrl coppia"(w1104) -> ()
                      n494 = local read "Array stato inverter freno"() -> (w1102:T1[])
                      n495 = Index Array(array=w1102, index=w1101) -> (element=w1103:T1)
                      n496 = Unbundle By Name(w1103) -> ("Ctrl velocità"=w1098:bool, "Ctrl coppia"=w1097:bool)
                      n497 = Not(x=w1098) -> (.not. x?=w1095:bool)
                      n498 = Not(x=w1097) -> (.not. x?=w1096:bool)
                      n499 = And(x=w1095, y=w1096) -> (x .and. y?=w1094:bool)
                      n500 = Select(t="Set controllo coppia", s=w1094, f=w1099) -> (s? t:f=w1093:string)
                    }
                    frame "Set controllo coppia" {
                      n501 = local read "Array stato inverter freno"() -> (w1109:T1[])
                      n502 = Index Array(array=w1109, index=w1108) -> (element=w1110:T1)
                      n503 = Unbundle By Name(w1110) -> ("Ctrl coppia"=w1107:bool)
                      n504 = local write "Ctrl coppia"(TRUE ("Ctrl coppia")) -> ()
                      n505 = Select(t="Set rif coppia", s=w1107, f=w1113) -> (s? t:f=w1112:string)
                    }
                    frame "Set rif coppia" {
                      n506 = case shown="\"Power [W]\"" w1122 {
                        tunnel: w1139 -> [w1140 _ _]
                        tunnel: [w1140 w1141 _] -> w1115
                        tunnel: w1138 -> [_ w1143 _]
                        tunnel: w1137 -> [_ w1142 _]
                        frame "Torque [Nm]", Default {
                        }
                        frame "Power [W]" {
                          n507 = call "Coppia da potenza.vi"("Pmecc W"=w1142, "RPM letti"=w1143) -> ("t"=w1141:dbl)  [unwired: 9 in]
                        }
                        frame "Speed [RPM]" {
                        }
                      }
                      n508 = local read "Array stato inverter freno"() -> (w1119:T1[])
                      n509 = Index Array(array=w1119, index=w1117) -> (element=w1120:T1)
                      n510 = Unbundle By Name(w1120) -> ("Rif AO coppia freno[Nm]"=w1118:dbl)
                      n511 = Divide(x=w1115, y=w1131) -> (x/y=w1133:dbl)
                      n512 = Multiply(x=w1133, y=100.0) -> (x*y=w1135:dbl)
                      n513 = In Range and Coerce(upper limit=100.0, x=w1135, lower limit=0.0) -> ()  [unwired: 2 out]
                      n514 = Absolute Value(x=w1115) -> (abs(x)=w1114:dbl)
                      n515 = Absolute Value(x=w1118) -> (abs(x)=w1116:dbl)
                      n516 = local write "Rif AO coppia freno [Nm]"(w1114) -> ()
                      n517 = Multiply(x=0.99, y=w1114) -> (x*y=w1127:dbl)
                      n518 = Multiply(x=1.01, y=w1114) -> (x*y=w1129:dbl)
                      n519 = In Range and Coerce(upper limit=w1129, x=w1116, lower limit=w1127) -> (In Range?=w1126:bool)  [unwired: 1 out]
                      n520 = Select(t="Togli blocco", s=w1126, f=w1125) -> (s? t:f=w1124:string)
                    }
                    frame "Togli blocco" {
                      n521 = global read "Global_All_Data.vi" "All Data"() -> (w1148:T11)
                      n522 = Unbundle By Name(w1148) -> ("Abilita AFE"=w1145:bool)
                      n523 = call "Set DO.vi"("Cluster SET DO"=T43 [{"DO"=enum."Comando azionam in blocco", "Value"=FALSE}]) -> ()  [unwired: 10 in, 1 out]
                      n524 = Select(t=w1147, s=w1145, f="Controllo azion reset" ("t")) -> (s? t:f=w1146:string)
                    }
                    frame "Controllo azion reset" {
                      n525 = global read "Global_All_Data.vi" "All Data"() -> (w1155:T11)
                      n526 = Unbundle By Name(w1155) -> ("MISURE ALL.STATO PLC 1.USCITE PLC.DO (bit).Reset allarmi"=w1154:bool)
                      n527 = call "Set DO.vi"("Cluster SET DO"=T43 [{"DO"=enum."Comando azionam reset", "Value"=TRUE}]) -> ()  [unwired: 10 in, 1 out]
                      n528 = Select(t="Togli reset", s=w1154, f=w1153) -> (s? t:f=w1152:string)
                    }
                    frame "Togli reset" {
                      n529 = global read "Global_All_Data.vi" "All Data"() -> (w1162:T11)
                      n530 = Unbundle By Name(w1162) -> ("MISURE ALL.STATO PLC 1.USCITE PLC.DO (bit).Reset allarmi"=w1161:bool)
                      n531 = call "Set DO.vi"("Cluster SET DO"=T43 [{"DO"=enum."Comando azionam reset", "Value"=FALSE}]) -> ()  [unwired: 10 in, 1 out]
                      n532 = Select(t=w1159, s=w1161, f="Fine imposta controllo coppia" ("t")) -> (s? t:f=w1160:string)
                    }
                    frame "Fine imposta controllo coppia" {
                      n533 = global write "Global CAMBIO CTRL FRENO.vi" "CAMBIO CTRL IN CORSO"(FALSE ("CAMBIO CTRL IN CORSO")) -> ()
                    }
                  }
                }
              }
              frame Enabled {
              }
            }
          }
        }
        n534 = case shown="False" w964 {
          tunnel: w965 -> [w1169 w1173]
          frame False {
            n535 = Enqueue Element(queue=w1169, element=cluster{"Status":string, "variant":variant} {"Status"="Passaggio velocità coppia", "variant"=variant}) -> ()  [unwired: 2 in, 3 out]
          }
          frame True {
            n536 = Flush Queue(queue=w1173) -> (queue out=w1171:refnum<queue>)  [unwired: 1 in, 2 out]
            n537 = Enqueue Element At Opposite End(queue=w1171, element=cluster{"Status":string, "variant":variant} {"Status"="REGOLA", "variant"=variant}) -> ()  [unwired: 2 in, 3 out]
          }
        }
      }
      frame "REGOLA" {
        n538 = Unbundle By Name(w1199) -> ("RPM"=w1174:dbl, "COPPIA"=w1196:dbl, "POTENZA"=w1193:dbl)
        n539 = Not A Number/Path/Refnum?(number/path/refnum=w1174) -> (NaN/Path/Refnum?=w1176:bool)
        n540 = Wait Until Next ms Multiple(millisecond multiple=w1183) -> ()  [unwired: 1 out]
        n541 = Select(t=0.0, s=w1176, f=w1174) -> (s? t:f=w1175:dbl)
        n542 = case shown="\"Power [W]\"" w1197 {
          selector: w1197 -> [_ _ w1372]
          tunnel: w1198 -> [w1269 w1337 w1366]
          tunnel: w1180 -> [_ _ w1359]
          tunnel: w1196 -> [w1255 _ w1365]
          tunnel: w1195 -> [w1244 w1297 w1370]
          tunnel: [w1230 w1297 w1362] -> w1194
          tunnel: w1175 -> [w1210 w1336 w1360]
          tunnel: w1193 -> [_ w1328 _]
          tunnel: w1192 -> [w1268 w1314 w1369]
          tunnel: [w1268 w1313 w1363] -> w1191
          tunnel: w1190 -> [w1266 w1334 w1361]
          tunnel: w1189 -> [w1265 w1333 w1368]
          tunnel: [w1265 w1333 w1367] -> w1188
          tunnel: w1183 -> [w1254 w1330 w1364]
          tunnel: w1185 -> [w1256 w1327 w1358]
          tunnel: [FALSE FALSE w1357] -> w1184
          tunnel: w1181 -> [w1228 w1287 w1356]
          tunnel: [_ _ w1354] -> w1179
          tunnel: w1178 -> [w1215 w1286 w1355]
          frame "Torque [Nm]", Default {
            n543 = local read "KW max banco"() -> (w1234:dbl)
            n544 = local read "Kw Max prova"() -> (w1239:dbl)
            n545 = Unbundle By Name(w1269) -> ("A max"=w1203:dbl, "Cmax"=w1200:dbl, "Compensa coppia residua"=w1253:T45, "Controllo coppia"=w1209:T46)
            n546 = local read "Rif AO coppia freno [Nm]"() -> (w1251:dbl)
            n547 = global read "Global control type freno.vi" "Value"() -> (w1205:T2)
            n548 = local read "Array stato inverter freno"() -> (w1229:T1[])
            n549 = local read "Abilita"() -> (w1250:bool)
            n550 = Not A Number/Path/Refnum?(number/path/refnum=w1210) -> (NaN/Path/Refnum?=w1211:bool)
            n551 = In Range and Coerce(upper limit=w1234, x=w1239, lower limit=0.0) -> (coerced(x)=w1236:dbl)  [unwired: 1 out]
            n552 = Equal?(x=w1205, y=T2."Corrente [A]") -> (x = y?=w1202:bool)
            n553 = Bundle By Name(cluster=w1209, "Precisione pid Nm"="Precisione pid Nm") -> (w1208:T46)
            n554 = Select(t=0.0, s=w1211, f=w1210) -> (s? t:f=w1213:dbl)
            n555 = Equal To 0?(x=w1236) -> (x = 0?=w1237:bool)
            n556 = Select(t=w1244, s=w1250, f=0.0) -> (s? t:f=w1249:dbl)
            n557 = Select(t=w1203, s=w1202, f=w1200) -> (s? t:f=w1201:dbl)
            n558 = Select(t=w1234, s=w1237, f=w1236) -> (s? t:f=w1235:dbl)
            n559 = In Range and Coerce(upper limit=w1201, x=w1249, lower limit=0.0) -> (coerced(x)=w1241:dbl, In Range?=w1240:bool)
            n560 = Multiply(x=w1235, y=1000.0) -> (x*y=w1246:dbl)
            n561 = Index Array(array=w1229, index=w1228) -> (element=w1227:T1)
            n562 = feedback-in #1(w1240) -> ()
            n563 = feedback #1() -> (w1243:bool)  [unwired: 1 in]
            n564 = call "Coppia da potenza.vi"("Pmecc W"=w1246, "RPM letti"=w1213) -> ()  [unwired: 9 in, 1 out]
            n565 = Unbundle By Name(w1208) -> ("Abilita pid"=w1221:bool)
            n566 = Not Equal?(x=w1240, y=w1243) -> (x != y?=w1242:bool)
            n567 = call "CONTROLLO RIFERIMENTO.vi"("Controllo"=w1208, "SET rampa"=w1241, "Lettura reale"=w1255, "New value?"=w1256, "RIFERIMENTO% in"=w1251, "SET pid"=w1241, "Valore MAX"=w1201, "Tciclo ms"=w1254, "output low pid =0"=FALSE) -> ("RIFERIMENTO% out"=w1231:dbl, "Stabile?"=→"C Stabile?":bool, "fine rampa"=→"fine rampa C":bool)  [unwired: 8 in]
            n568 = case shown="True" w1242 {
              tunnel: w1244 -> [w1270 w1274]
              tunnel: [w1270 w1273] -> w1230
              tunnel: w1240 -> [_ w1272]
              tunnel: w1241 -> [_ w1271]
              frame False {
              }
              frame True {
                n569 = case shown="False" w1272 {
                  tunnel: w1274 -> [_ w1276]
                  tunnel: [w1275 w1276] -> w1273
                  tunnel: w1271 -> [w1275 _]
                  frame False {
                    n570 = property on="Set" class="DigNum (strict)"("Value"=w1275) -> ()  [unwired: 2 in, 2 out]
                  }
                  frame True {
                  }
                }
              }
            }
            n571 = local read "Compensazione velocità"() -> (w1214:bool)
            n572 = Unbundle By Name(w1253) -> ("C residua [Nm]"=w1258:dbl)
            n573 = Less Or Equal To 0?(x=w1231) -> (x <= 0?=w1233:bool)
            n574 = Greater?(x=w1213, y=500.0) -> (0:w1216:bool)
            n575 = Unbundle By Name(w1227) -> ("Running"=w1226:bool)
            n576 = Select(t=0.0 ("f"), s=w1233, f=w1231) -> (s? t:f=w1222:dbl)
            n577 = Equal To 0?(x=w1222) -> (x = 0?=w1220:bool)
            n578 = Less?(x=w1230, y=w1258) -> (x < y?=w1267:bool)
            n579 = Divide(x=w1222, y=w1201) -> (x/y=w1264:dbl)
            n580 = Select(t=w1220, s=w1221, f=TRUE) -> (s? t:f=w1219:bool)
            n581 = And(x=w1215, y=w1216) -> (x .and. y?=w1217:bool)
            n582 = Multiply(x=w1264, y=100.0) -> (x*y=w1262:dbl)
            n583 = Compound Arithmetic op=AND(w1217, w1267, w1214, w1226, w1219) -> (w1223:bool)
            n584 = In Range and Coerce(upper limit=100.0, x=w1262, lower limit=0.0) -> ()  [unwired: 2 out]
            n585 = case shown="True" w1223 {
              tunnel: w1266 -> [w1277 w1280]
              frame False {
                n586 = Enqueue Element(queue=w1277, element=cluster{"Status":string, "variant":variant} {"Status"="REGOLA", "variant"=variant}) -> ()  [unwired: 2 in, 3 out]
              }
              frame True {
                n587 = Flush Queue(queue=w1280) -> (queue out=w1279:refnum<queue>)  [unwired: 1 in, 2 out]
                n588 = Enqueue Element(queue=w1279, element=cluster{"Status":string, "variant":variant} {"Status"="Passaggio coppia velocità", "variant"=variant}) -> ()  [unwired: 2 in, 3 out]
              }
            }
            n589 = local write "Rif AO coppia freno [Nm]"(w1222) -> ()
            n590 = local write "Rif AO vel [RPM]"("Rif % AO RPM") -> ()
          }
          frame "Power [W]" {
            # "Condizione per passare al controllo di velocità (compensazione coppia residua): il setpoint deve essere inferiore della coppia residua, e se il pid è abilitato\naspettare che lil rif di coppia vada a 0 in modo da essere sicuri che non sia possibile raggiungere la potenza impostata agendo solo sul rif di coppia"
            n591 = local read "KW max banco"() -> (w1304:dbl)
            n592 = local read "Kw Max prova"() -> (w1308:dbl)
            n593 = Unbundle By Name(w1337) -> ("Cmax"=w1319:dbl, "Compensa coppia residua"=w1329:T45, "Controllo potenza"=w1284:T47)
            n594 = local read "Abilita"() -> (w1323:bool)
            n595 = In Range and Coerce(upper limit=w1304, x=w1308, lower limit=0.0) -> (coerced(x)=w1303:dbl)  [unwired: 1 out]
            n596 = feedback #2() -> (w1325:dbl)  [unwired: 1 in]
            n597 = local read "Array stato inverter freno"() -> (w1290:T1[])
            n598 = Select(t=w1314, s=w1323, f=0.0) -> (s? t:f=w1315:dbl)
            n599 = Equal To 0?(x=w1303) -> (x = 0?=w1305:bool)
            n600 = Select(t=w1304, s=w1305, f=w1303) -> (s? t:f=w1302:dbl)
            n601 = local read "Rif AO coppia freno [Nm]"() -> (w1324:dbl)
            n602 = In Range and Coerce(upper limit=w1302, x=w1315, lower limit=0.0) -> (coerced(x)=w1310:dbl, In Range?=w1309:bool)
            n603 = Bundle By Name(cluster=w1284, "Precisione pid W"="Precisione pid W") -> (w1283:T47)
            n604 = feedback-in #3(w1309) -> ()
            n605 = feedback #3() -> (w1312:bool)  [unwired: 1 in]
            n606 = Index Array(array=w1290, index=w1287) -> (element=w1289:T1)
            n607 = Not Equal?(x=w1309, y=w1312) -> (x != y?=w1311:bool)
            n608 = Multiply(x=1000.0, y=w1310) -> (x*y=w1318:dbl)
            n609 = case shown="True" w1327 {
              tunnel: w1336 -> [_ w1348]
              tunnel: [w1345 w1347] -> w1326
              tunnel: w1318 -> [_ w1346]
              tunnel: w1325 -> [w1345 _]
              frame False {
              }
              frame True {
                n610 = call "Coppia da potenza.vi"("Pmecc W"=w1346, "RPM letti"=w1348) -> ("t"=w1347:dbl)  [unwired: 9 in]
              }
            }
            n611 = feedback-in #2(w1326) -> ()
            n612 = Unbundle By Name(w1289) -> ("Running"=w1288:bool)
            n613 = Unbundle By Name(w1329) -> ("C residua [Nm]"=w1332:dbl)
            n614 = Unbundle By Name(w1284) -> ("Abilita pid"=w1294:bool)
            n615 = call "CONTROLLO RIFERIMENTO.vi"("Controllo"=w1283, "SET rampa"=w1326, "Lettura reale"=w1328, "New value?"=w1327, "RIFERIMENTO% in"=w1324, "SET pid"=w1318, "Valore MAX"=w1319, "Tciclo ms"=w1330, "output low pid =0"=FALSE) -> ("RIFERIMENTO% out"=w1299:dbl, "Stabile?"=w1321:bool, "fine rampa"=w1296:bool)  [unwired: 8 in]
            n616 = case shown="True" w1311 {
              tunnel: w1309 -> [_ w1342]
              tunnel: w1314 -> [w1338 w1341]
              tunnel: [w1338 w1340] -> w1313
              tunnel: w1310 -> [_ w1339]
              frame False {
              }
              frame True {
                n617 = case shown="False" w1342 {
                  tunnel: w1341 -> [_ w1344]
                  tunnel: [w1343 w1344] -> w1340
                  tunnel: w1339 -> [w1343 _]
                  frame False {
                    n618 = property on="Set" class="DigNum (strict)"("Value"=w1343) -> ()  [unwired: 2 in, 2 out]
                  }
                  frame True {
                  }
                }
              }
            }
            n619 = Less Or Equal To 0?(x=w1299) -> (x <= 0?=w1301:bool)
            n620 = Select(t=0.0 ("f"), s=w1301, f=w1299) -> (s? t:f=w1295:dbl)
            n621 = Equal To 0?(x=w1295) -> (x = 0?=w1293:bool)
            n622 = Less?(x=w1295, y=w1332) -> (x < y?=w1335:bool)
            n623 = local write "fine rampa C"(w1296) -> ()
            n624 = And(x=w1321, y=w1296) -> (x .and. y?=→"P Stabile?":bool)
            n625 = Select(t=w1293, s=w1294, f=TRUE) -> (s? t:f=w1292:bool)
            n626 = Compound Arithmetic op=AND(w1286, w1288, w1335, "Compensazione velocità", w1296, w1292) -> (w1298:bool)
            n627 = local write "Rif AO coppia freno [Nm]"(w1295) -> ()
            n628 = case shown="True" w1298 {
              tunnel: w1334 -> [w1349 w1352]
              frame False {
                n629 = Enqueue Element(queue=w1349, element=cluster{"Status":string, "variant":variant} {"Status"="REGOLA", "variant"=variant}) -> ()  [unwired: 2 in, 3 out]
              }
              frame True {
                n630 = Flush Queue(queue=w1352) -> (queue out=w1351:refnum<queue>)  [unwired: 1 in, 2 out]
                n631 = Enqueue Element(queue=w1351, element=cluster{"Status":string, "variant":variant} {"Status"="Passaggio coppia velocità", "variant"=variant}) -> ()  [unwired: 2 in, 3 out]
              }
            }
          }
          frame "Speed [RPM]" {
            n632 = Equal?(x=w1372, y=w1359) -> (x = y?=w1371:bool)
            n633 = case shown="False" w1371 {
              tunnel: w1370 -> [w1408 w1445]
              tunnel: w1369 -> [w1411 w1446]
              tunnel: w1368 -> [w1398 w1428]
              tunnel: [w1398 w1428] -> w1367
              tunnel: w1366 -> [w1422 w1442]
              tunnel: w1365 -> [w1407 _]
              tunnel: w1364 -> [w1403 w1437]
              tunnel: [w1411 w1446] -> w1363
              tunnel: [w1408 w1445] -> w1362
              tunnel: w1361 -> [w1415 w1443]
              tunnel: w1360 -> [w1412 w1439]
              tunnel: w1359 -> [w1409 _]
              tunnel: w1358 -> [_ w1440]
              tunnel: [TRUE _] -> w1357
              tunnel: w1356 -> [w1382 _]
              tunnel: w1355 -> [w1378 _]
              tunnel: [TRUE _] -> w1354
              frame False {
                w1386 = FALSE ("f")
                # "New value in\nmodo che se\ntorno al\ncontrollo in\ncoppia o\npotenza,\nriparto con la\nregolazione dal\nsetpoint di C o P"
                # "PORTATI ALLA COPPIA IMPOSTATA VARIANDO I GIRI"
                n634 = Unbundle By Name(w1422) -> ("Rpm max"=w1406:dbl, "Compensa coppia residua"=w1413:T45, "Compensa coppia residua.Max%pid"=w1400:i32)
                n635 = local read "Array stato inverter freno"() -> (w1384:T1[])
                n636 = Multiply(x=w1411, y=1000.0) -> (x*y=w1395:dbl)
                n637 = Equal?(x=w1409, y=T2."Torque [Nm]" ("Value")) -> (x = y?=w1390:bool)
                n638 = call "Coppia da potenza.vi"("Pmecc W"=w1395, "RPM letti"=w1412) -> ("t"=w1410:dbl)  [unwired: 9 in]
                n639 = Select(t=w1408, s=w1390, f=w1410) -> (s? t:f=w1392:dbl)
                n640 = Divide(x=w1403, y=1000.0) -> (x/y=w1402:dbl)
                n641 = Index Array(array=w1384, index=w1382) -> (element=w1383:T1)
                n642 = Unbundle By Name(w1413) -> ("PID gains C-RPM"=w1405:T48, "C precision [Nm]"=w1404:dbl)
                n643 = Unbundle By Name(w1383) -> ("Running"=w1381:bool)
                n644 = local read "Compensazione velocità"() -> (w1377:bool)
                n645 = Not(x=w1378) -> (.not. x?=w1374:bool)
                n646 = Unbundle By Name(w1413) -> ("C isteresi [Nm]"=w1414:dbl)
                n647 = Not(x=w1381) -> (.not. x?=w1380:bool)
                n648 = call "PID COPPIA.vi"("setpoint"=w1392, "Max"=w1406, "%max"=w1400, "output low pid =0"=FALSE, "process variable"=w1407, "PID gains"=w1405, "dt (s)"=w1402, "Precisione"=w1404, "Abilita pid"=TRUE, "Escludi init new value"=TRUE) -> ("output"=w1399:dbl, "Stabile?"=w1389:bool)  [unwired: 4 in]
                n649 = Subtract(x=w1398, y=w1399) -> (x-y=w1397:dbl)
                n650 = Select(t=w1386, s=w1390, f=w1389) -> (s? t:f=w1388:bool)
                n651 = Select(t=w1389, s=w1390, f=w1386) -> (s? t:f=w1387:bool)
                n652 = Not(x=w1377) -> (.not. x?=w1376:bool)
                n653 = Greater?(x=w1392, y=w1414) -> (0:w1385:bool)
                n654 = Divide(x=w1397, y=w1406) -> (x/y=w1418:dbl)
                n655 = local write "C Stabile?"(w1387) -> ()
                n656 = local write "P Stabile?"(w1388) -> ()
                n657 = Multiply(x=w1418, y=100.0) -> (x*y=w1420:dbl)
                n658 = Compound Arithmetic op=OR(w1374, w1380, w1385, w1376) -> (w1379:bool)
                n659 = case shown="True" w1379 {
                  tunnel: w1415 -> [w1423 w1426]
                  frame False {
                    n660 = Enqueue Element(queue=w1423, element=cluster{"Status":string, "variant":variant} {"Status"="REGOLA", "variant"=variant}) -> ()  [unwired: 2 in, 3 out]
                  }
                  frame True {
                    n661 = Flush Queue(queue=w1426) -> (queue out=w1425:refnum<queue>)  [unwired: 1 in, 2 out]
                    n662 = Enqueue Element(queue=w1425, element=cluster{"Status":string, "variant":variant} {"Status"="Passaggio velocità coppia", "variant"=variant}) -> ()  [unwired: 2 in, 3 out]
                  }
                }
                n663 = In Range and Coerce(upper limit=100.0, x=w1420, lower limit=0.0) -> ()  [unwired: 2 out]
                n664 = local write "Rif AO vel [RPM]"(w1397) -> ()
              }
              frame True {
                n665 = local read "Abilita"() -> (w1432:bool)
                n666 = Unbundle By Name(w1442) -> ("Controllo RPM"=w1441:T49)
                n667 = Unbundle By Name(w1442) -> ("Rpm max"=w1438:dbl)
                n668 = Less Than 0?(x=w1428) -> ()  [unwired: 1 out]
                n669 = local read "Rif AO vel [RPM]"() -> (w1429:dbl)
                n670 = Select(t=w1428, s=w1432, f=0.0) -> (s? t:f=w1431:dbl)
                n671 = Absolute Value(x=w1431) -> (abs(x)=w1433:dbl)
                n672 = call "CONTROLLO RIFERIMENTO.vi"("Controllo"=w1441, "SET rampa"=w1433, "Lettura reale"=w1439, "New value?"=w1440, "RIFERIMENTO% in"=w1429, "SET pid"=w1433, "Valore MAX"=w1438, "Tciclo ms"=w1437) -> ("RIFERIMENTO% out"=w1435:dbl, "Stabile?"=→"Rpm stabile":bool, "fine rampa"=→"fine rampa rpm":bool)  [unwired: 9 in]
                n673 = local write "Rif AO vel [RPM]"(w1435) -> ()
                n674 = Enqueue Element(queue=w1443, element=cluster{"Status":string, "variant":variant} {"Status"="REGOLA", "variant"=variant}) -> ()  [unwired: 2 in, 3 out]
              }
            }
          }
        }
        "Comp." <- w1179
      }
      frame "EXIT" {
        w1447 = TRUE ("stop")
        n675 = property on="EXIT" class="Bool (strict)"("Val(Sgnl)"=w1447) -> ()  [unwired: 2 in, 2 out]
        n676 = local write "stop"(w1447) -> ()
      }
    }
    "Stato comandi" <- w249
    "rpm->C" <- w257
    "C->rpm" <- w247
    "Numeric" <- w255
    "Controllo effettivo" <- w269
    "Controllo desiderato" <- w265
    "Freno selezionato" <- w253
  }
  n677 = while {
    tunnel: w10 -> [w1460]
    stop <- w1459 stop-if-true
    n678 = event shown="[2] \"Gestione freno.Start\\stop\", \"Gestione freno.Status\", \"Gestione freno.PID\", \"Gestione freno.Abilita\", \"Gestione freno.Status ref\", \"Gestione freno.Control.Set\", \"Gestione freno.Control.Inverti senso di rotazione\": Value Change" {
      selector: _ -> [_ _ _ _ _ _ _]
      dyn-events: _ -> [_ _ _ _ _ _ _]
      timeout: _ -> [_ _ _ _ _ _ _]
      tunnel: w1460 -> [_ _ w1471 w1477 w1495 _ w1504]
      tunnel: [_ _ _ _ _ _ TRUE] -> w1459
      event Timeout {
        n679 = event-data() -> ()  [unwired: 1 in, 3 out]
      }
      event "Salva config freni": Value Change {
        n680 = event-data() -> ()  [unwired: 1 in, 6 out]
        n681 = local read "ARRAY IMPOSTAZIONI INV.FRENI"() -> (w1461:T4[])
        n682 = call <vilib>:"Application Directory.vi"() -> ("Application Directory"=w1467:path)
        n683 = Build Path(base path=w1467, name or relative path="Settings\\Configurazione_Freni") -> (appended path=w1468:path)
        n684 = Open/Create/Replace File(file path (use dialog)=w1468, operation (0:open)=T41."replace or create") -> (refnum out=w1463:refnum<file>, error out=w1464:errorcluster)  [unwired: 4 in, 1 out]
        n685 = Write to Binary File(file (use dialog)=w1463, data=w1461, error in=w1464) -> (refnum out=w1465:refnum<file>, error out=w1466:errorcluster)  [unwired: 3 in, 1 out]
        n686 = Close File(refnum=w1465, error in=w1466) -> ()  [unwired: 2 out]
      }
      event Value Change {
        n687 = event-data() -> ()  [unwired: 1 in, 6 out]
        n688 = local read "Gestione freno"() -> (w1470:T3)
        n689 = Bundle By Name(cluster=cluster{"Status":string, "variant":variant} {"Status"="AGGIORNA COMANDI FRENO", "variant"=variant}, "variant"=w1470) -> (w1472:cluster{"Status":string, "variant":variant})
        n690 = Enqueue Element At Opposite End(queue=w1471, element=w1472) -> ()  [unwired: 2 in, 3 out]
      }
      event Value Change {
        n691 = event-data() -> ("NewVal"=w1478:T2)  [unwired: 1 in]
        n692 = case shown="\"Torque [Nm]\", Default" w1478 {
          tunnel: [w1485 w1487 w1488 w1491] -> w1480
          tunnel: [w1484 w1486 w1489 w1490] -> w1482
          frame "Torque [Nm]", Default {
            n693 = local read "Nm max Banco 2"() -> (w1484:dbl)
            n694 = local read "Nm max Banco 1"() -> (w1485:dbl)
          }
          frame "Power [W]" {
            n695 = local read "KW max Banco 2"() -> (w1486:dbl)
            n696 = local read "KW max Banco 1"() -> (w1487:dbl)
          }
          frame "Speed [RPM]" {
            n697 = local read "RPM max Banco 2"() -> (w1489:dbl)
            n698 = local read "RPM max Banco 1"() -> (w1488:dbl)
          }
          frame "Corrente [A]" {
            n699 = local read "A max Banco 1"() -> (w1491:dbl)
            n700 = local read "A max Banco 2"() -> (w1490:dbl)
          }
        }
        n701 = global read "BenchSelector.vi" "Bench Selector"() -> (w1481:bool)
        n702 = local read "Gestione freno"() -> (w1475:T3)
        n703 = Select(t=w1482, s=w1481, f=w1480) -> (s? t:f=w1483:dbl)
        n704 = property on="Set" class="DigNum (strict)"("Maximum"=w1483, "Minimum"=0.0 ("Data Entry Limits:Minimum")) -> ()  [unwired: 2 in, 2 out]
        n705 = Bundle By Name(cluster=cluster{"Status":string, "variant":variant} {"Status"="AGGIORNA COMANDI FRENO", "variant"=variant}, "variant"=w1475) -> (w1474:cluster{"Status":string, "variant":variant})
        n706 = Enqueue Element(queue=w1477, element=w1474) -> ()  [unwired: 2 in, 3 out]
      }
      event "ARRAY IMPOSTAZIONI INV.FRENI": Value Change {
        n707 = event-data() -> ()  [unwired: 1 in, 6 out]
        n708 = Bundle By Name(cluster=T5 {"Message"="AGGIORNA SETTINGS FRENI", "Message Data"=variant} ("element"), "Message Data"="ARRAY IMPOSTAZIONI INV.FRENI") -> (w1493:T5)
        n709 = Enqueue Element(queue=w1495, element=w1493) -> ()  [unwired: 2 in, 3 out]
      }
      event "rif vel": Value Change {
        n710 = event-data() -> ()  [unwired: 1 in, 6 out]
        n711 = Two Button Dialog(message="---- ATTENZIONE ---\n\nModificare il valore di riferimento\ndi velocità per le modalità\nCOPPIA e POTENZA ?") -> (T button?=w1497:bool)  [unwired: 2 in]
        n712 = case shown="True" w1497 {
          frame False {
          }
          frame True {
            n713 = call "Prompt User for Input"() -> ("Rif. velocità [RPM]"=w1500:dbl, "OK"=w1501:bool)  [unwired: 17 in, 1 out]
            n714 = Select(t=w1500, s=w1501, f=0.0) -> (s? t:f=w1499:dbl)
            n715 = local write "Rif % AO RPM"(w1499) -> ()
          }
        }
      }
      event "EXIT": Value Change {
        n716 = event-data() -> ()  [unwired: 1 in, 6 out]
        n717 = Enqueue Element(queue=w1504, element=T5 {"Message"="EXIT", "Message Data"=variant}) -> ()  [unwired: 2 in, 3 out]
      }
    }
  }
